vi "SIAM_test_Standalone-Dev.vi"() -> ()   [LabVIEW 2011]
doc: "Tool for TILL ID SIAM hardware test."
uses:
  SIAM_command.ctl
  SIAM-axis.ctl
  SIAM-send.ctl
panel:
  out "Connected":bool
  in  "Format":enum16{"Hex", "dez", "Ascii", "dez16s"}(ring)
  in  "Run":bool
  in  "Clear":bool
  in  "return":string
  in  "Registerkarte":T1(tab)
  in  "connect":bool caption="disconnect"
  in  "ScaleConst":T3(array[cluster])=[{"Axis-Ring"=104857665, "Scale"=500.0, "Offset"=1000000.0, "HW min"=0.0, "HW max"=4000.0, "max a"=inf, "max v"=inf, "units"="µm"}, {"Axis-Ring"=102760513, "Scale"=1.0, "Offset"=0.0, "HW min"=-32000.0, "HW max"=32000.0, "max a"=5.0, "max v"=inf, "units"="c"}, {"Axis-Ring"=101711937, "Scale"=1.0, "Offset"=0.0, "HW min"=-32000.0, "HW max"=32000.0, "max a"=0.02, "max v"=inf, "units"="c"}, {"Axis-Ring"=16777217, "Scale"=51200.0, "Offset"=100.0, "HW min"=0.0, "HW max"=5500000.0, "max a"=inf, "max v"=20.0, "units"="mm"}, {"Axis-Ring"=17825793, "Scale"=51200.0, "Offset"=100.0, "HW min"=0.0, "HW max"=3700000.0, "max a"=inf, "max v"=20.0, "units"="mm"}, {"Axis-Ring"=19922945, "Scale"=153600.0, "Offset"=146600.0, "HW min"=0.0, "HW max"=614400.0, "max a"=inf, "max v"=1.0, "units"="Pos"}, {"Axis-Ring"=20971521, "Scale"=25000.1, "Offset"=641.0, "HW min"=0.0, "HW max"=124721.0, "max a"=inf, "max v"=1.0, "units"="Pos"}, {"Axis-Ring"=22020097, "Scale"=1.0, "Offset"=0.0, "HW min"=0.0, "HW max"=51200.0, "max a"=inf, "max v"=inf, "units"="counts"}, {"Axis-Ring"=23068673, "Scale"=10240.0, "Offset"=0.0, "HW min"=0.0, "HW max"=51200.0, "max a"=inf, "max v"=inf, "units"="Pos"}, {"Axis-Ring"=24117249, "Scale"=1.0, "Offset"=0.0, "HW min"=0.0, "HW max"=51200.0, "max a"=inf, "max v"=inf, "units"="counts"}, {"Axis-Ring"=2684354561, "Scale"=1.0, "Offset"=0.0, "HW min"=0.0, "HW max"=65636.0, "max a"=inf, "max v"=inf, "units"="counts"}, {"Axis-Ring"=2685403137, "Scale"=1.0, "Offset"=0.0, "HW min"=0.0, "HW max"=65636.0, "max a"=inf, "max v"=inf, "units"="counts"}, {"Axis-Ring"=2686451713, "Scale"=1.0, "Offset"=0.0, "HW min"=0.0, "HW max"=65636.0, "max a"=inf, "max v"=inf, "units"="counts"}, {"Axis-Ring"=2687500289, "Scale"=1.0, "Offset"=0.0, "HW min"=0.0, "HW max"=65636.0, "max a"=inf, "max v"=inf, "units"="counts"}, {"Axis-Ring"=2688548865, "Scale"=1.0, "Offset"=0.0, "HW min"=0.0, "HW max"=65636.0, "max a"=inf, "max v"=inf, "units"="counts"}, {"Axis-Ring"=2689597441, "Scale"=1.0, "Offset"=1.0, "HW min"=0.0, "HW max"=65636.0, "max a"=inf, "max v"=inf, "units"="counts"}, {"Axis-Ring"=2690646017, "Scale"=1.0, "Offset"=1.0, "HW min"=0.0, "HW max"=65636.0, "max a"=inf, "max v"=inf, "units"="counts"}, {"Axis-Ring"=2691694593, "Scale"=1.0, "Offset"=1.0, "HW min"=0.0, "HW max"=65636.0, "max a"=inf, "max v"=inf, "units"="counts"}, {"Axis-Ring"=2701131777, "Scale"=1.0, "Offset"=1.0, "HW min"=0.0, "HW max"=65636.0, "max a"=inf, "max v"=inf, "units"="counts"}, {"Axis-Ring"=2702180353, "Scale"=1.0, "Offset"=1.0, "HW min"=0.0, "HW max"=65636.0, "max a"=inf, "max v"=inf, "units"="counts"}, {"Axis-Ring"=2703228929, "Scale"=1.0, "Offset"=1.0, "HW min"=0.0, "HW max"=65636.0, "max a"=inf, "max v"=inf, "units"="counts"}, {"Axis-Ring"=2704277505, "Scale"=1.0, "Offset"=1.0, "HW min"=0.0, "HW max"=65636.0, "max a"=inf, "max v"=inf, "units"="counts"}, {"Axis-Ring"=2717908993, "Scale"=1.0, "Offset"=1.0, "HW min"=0.0, "HW max"=65636.0, "max a"=inf, "max v"=inf, "units"="counts"}, {"Axis-Ring"=2718957569, "Scale"=1.0, "Offset"=1.0, "HW min"=0.0, "HW max"=65636.0, "max a"=inf, "max v"=inf, "units"="counts"}, {"Axis-Ring"=2720006145, "Scale"=1.0, "Offset"=1.0, "HW min"=0.0, "HW max"=65636.0, "max a"=inf, "max v"=inf, "units"="counts"}, {"Axis-Ring"=2721054721, "Scale"=1.0, "Offset"=1.0, "HW min"=0.0, "HW max"=65636.0, "max a"=inf, "max v"=inf, "units"="counts"}, {"Axis-Ring"=67108865, "Scale"=1.0, "Offset"=1.0, "HW min"=100000.0, "HW max"=200000.0, "max a"=inf, "max v"=inf, "units"="counts"}, {"Axis-Ring"=68157441, "Scale"=1.0, "Offset"=1.0, "HW min"=100000.0, "HW max"=200000.0, "max a"=inf, "max v"=inf, "units"="counts"}] {"Axis-Ring" items=["255Axis"=16777217, "1-Axis"=17825793, "2-Axis"=18874369, "3-Axis"=19922945, "4-Axis"=20971521, "5-Axis"=22020097, "6-Axis"=23068673, "7-Axis"=24117249, "LED365"=2684354561, "LED385"=2685403137, "LED440"=2686451713, "LED470"=2687500289, "LED510"=2688548865, "LED540"=2689597441, "LED590"=2690646017, "LED640"=2691694593, "DurchR"=2701131777, "DurchG"=2702180353, "DurchB"=2703228929, "AF"=2704277505, "Laser0"=2717908993, "Laser1"=2718957569, "Laser2"=2720006145, "Laser3"=2721054721, "Servo0"=67108865, "Servo1"=68157441, "Servo2"=69206017, "Servo3"=70254593, "0-TMSI"=100663361, "1-TMSI"=101711937, "x-tmsi"=102760513, "y-tmsi"=103809089, "z-tmsi"=104857665, "orca1"=503316481, "orca2"=503316482, "orca3"=503316483, "orca4"=503316484, ""=0]}
  in  "instrument name":string="Till-X-3"
  in  "remote port":u16=3
  in  "address":string="192.168.99.3"
  out "connect error":errorcluster
  in  "Read":bool
  in  "Axis":T4={"Linear"={"Axis-Ring"=17825793, "Position"=824034}, "Linear"={"Axis-Ring"=18874369, "Position"=463519}, "Linear 2"={"Axis-Ring"=19922945, "Position"=689614}, "Linear 3"={"Axis-Ring"=101711937, "Position"=0}, "Linear"={"Axis-Ring"=102760513, "Position"=0}, "Linear 4"={"Axis-Ring"=2684354561, "Position"=0}, "Linear 5"={"Axis-Ring"=2685403137, "Position"=0}, "Linear 6"={"Axis-Ring"=2687500289, "Position"=0}, "Linear 7"={"Axis-Ring"=2691694593, "Position"=0}, "Linear 8"={"Axis-Ring"=2701131777, "Position"=0}, "Linear 9"={"Axis-Ring"=2717908993, "Position"=0}, "Linear 10"={"Axis-Ring"=2718957569, "Position"=0}, "Linear 11"={"Axis-Ring"=2720006145, "Position"=0}, "Linear 12"={"Axis-Ring"=503316482, "Position"=0}, "Linear 13"={"Axis-Ring"=67108865, "Position"=150000}} {"Linear 13"."Axis-Ring" items=["X-Axis"=16777217, "Y-Axis"=17825793, "Obj"=19922945, "Filter"=20971521, "Trans"=22020097, "FRET"=23068673, "SI"=24117249, "LED365"=2684354561, "LED385"=2685403137, "LED440"=2686451713, "LED470"=2687500289, "LED510"=2688548865, "LED540"=2689597441, "LED590"=2690646017, "LED640"=2691694593, "DurchR"=2701131777, "DurchG"=2702180353, "DurchB"=2703228929, "AF"=2704277505, "Laser0"=2717908993, "Laser1"=2718957569, "Laser2"=2720006145, "Laser3"=2721054721, "Servo0"=67108865, "Servo1"=68157441, "Servo2"=69206017, "Servo3"=70254593]; "Linear 13"."Position" scale=100000.0..200000.0; "Linear 12"."Axis-Ring" items=["255Axis"=16777217, "1-Axis"=17825793, "2-Axis"=18874369, "3-Axis"=19922945, "4-Axis"=20971521, "5-Axis"=22020097, "6-Axis"=23068673, "7-Axis"=24117249, "LED365"=2684354561, "LED385"=2685403137, "LED440"=2686451713, "LED470"=2687500289, "LED510"=2688548865, "LED540"=2689597441, "LED590"=2690646017, "LED640"=2691694593, "DurchR"=2701131777, "DurchG"=2702180353, "DurchB"=2703228929, "AF"=2704277505, "Laser0"=2717908993, "Laser1"=2718957569, "Laser2"=2720006145, "Laser3"=2721054721, "Servo0"=67108865, "Servo1"=68157441, "Servo2"=69206017, "Servo3"=70254593, "0-TMSI"=100663361, "1-TMSI"=101711937, "x-tmsi"=102760513, "y-tmsi"=103809089, "z-tmsi"=104857665, "orca1"=503316481, "orca2"=503316482, "orca3"=503316483, "orca4"=503316484, ""=0]; "Linear 12"."Position" scale=0.0..100.0; "Linear 11"."Axis-Ring" items=["255Axis"=16777217, "1-Axis"=17825793, "2-Axis"=18874369, "3-Axis"=19922945, "4-Axis"=20971521, "5-Axis"=22020097, "6-Axis"=23068673, "7-Axis"=24117249, "LED365"=2684354561, "LED385"=2685403137, "LED440"=2686451713, "LED470"=2687500289, "LED510"=2688548865, "LED540"=2689597441, "LED590"=2690646017, "LED640"=2691694593, "DurchR"=2701131777, "DurchG"=2702180353, "DurchB"=2703228929, "AF"=2704277505, "Laser0"=2717908993, "Laser1"=2718957569, "Laser2"=2720006145, "Laser3"=2721054721, "Servo0"=67108865, "Servo1"=68157441, "Servo2"=69206017, "Servo3"=70254593, "0-TMSI"=100663361, "1-TMSI"=101711937, "x-tmsi"=102760513, "y-tmsi"=103809089, "z-tmsi"=104857665, "orca1"=503316481, "orca2"=503316482, "orca3"=503316483, "orca4"=503316484, ""=0]; "Linear 11"."Position" scale=0.0..65000.0; "Linear 10"."Axis-Ring" items=["255Axis"=16777217, "1-Axis"=17825793, "2-Axis"=18874369, "3-Axis"=19922945, "4-Axis"=20971521, "5-Axis"=22020097, "6-Axis"=23068673, "7-Axis"=24117249, "LED365"=2684354561, "LED385"=2685403137, "LED440"=2686451713, "LED470"=2687500289, "LED510"=2688548865, "LED540"=2689597441, "LED590"=2690646017, "LED640"=2691694593, "DurchR"=2701131777, "DurchG"=2702180353, "DurchB"=2703228929, "AF"=2704277505, "Laser0"=2717908993, "Laser1"=2718957569, "Laser2"=2720006145, "Laser3"=2721054721, "Servo0"=67108865, "Servo1"=68157441, "Servo2"=69206017, "Servo3"=70254593, "0-TMSI"=100663361, "1-TMSI"=101711937, "x-tmsi"=102760513, "y-tmsi"=103809089, "z-tmsi"=104857665, "orca1"=503316481, "orca2"=503316482, "orca3"=503316483, "orca4"=503316484, ""=0]; "Linear 10"."Position" scale=0.0..65000.0; "Linear 9"."Axis-Ring" items=["255Axis"=16777217, "1-Axis"=17825793, "2-Axis"=18874369, "3-Axis"=19922945, "4-Axis"=20971521, "5-Axis"=22020097, "6-Axis"=23068673, "7-Axis"=24117249, "LED365"=2684354561, "LED385"=2685403137, "LED440"=2686451713, "LED470"=2687500289, "LED510"=2688548865, "LED540"=2689597441, "LED590"=2690646017, "LED640"=2691694593, "DurchR"=2701131777, "DurchG"=2702180353, "DurchB"=2703228929, "AF"=2704277505, "Laser0"=2717908993, "Laser1"=2718957569, "Laser2"=2720006145, "Laser3"=2721054721, "Servo0"=67108865, "Servo1"=68157441, "Servo2"=69206017, "Servo3"=70254593, "0-TMSI"=100663361, "1-TMSI"=101711937, "x-tmsi"=102760513, "y-tmsi"=103809089, "z-tmsi"=104857665, "orca1"=503316481, "orca2"=503316482, "orca3"=503316483, "orca4"=503316484, ""=0]; "Linear 9"."Position" scale=0.0..65000.0; "Linear 8"."Axis-Ring" items=["255Axis"=16777217, "1-Axis"=17825793, "2-Axis"=18874369, "3-Axis"=19922945, "4-Axis"=20971521, "5-Axis"=22020097, "6-Axis"=23068673, "7-Axis"=24117249, "LED365"=2684354561, "LED385"=2685403137, "LED440"=2686451713, "LED470"=2687500289, "LED510"=2688548865, "LED540"=2689597441, "LED590"=2690646017, "LED640"=2691694593, "DurchR"=2701131777, "DurchG"=2702180353, "DurchB"=2703228929, "AF"=2704277505, "Laser0"=2717908993, "Laser1"=2718957569, "Laser2"=2720006145, "Laser3"=2721054721, "Servo0"=67108865, "Servo1"=68157441, "Servo2"=69206017, "Servo3"=70254593, "0-TMSI"=100663361, "1-TMSI"=101711937, "x-tmsi"=102760513, "y-tmsi"=103809089, "z-tmsi"=104857665, "orca1"=503316481, "orca2"=503316482, "orca3"=503316483, "orca4"=503316484, ""=0]; "Linear 8"."Position" scale=0.0..65000.0; "Linear 7"."Axis-Ring" items=["255Axis"=16777217, "1-Axis"=17825793, "2-Axis"=18874369, "3-Axis"=19922945, "4-Axis"=20971521, "5-Axis"=22020097, "6-Axis"=23068673, "7-Axis"=24117249, "LED365"=2684354561, "LED385"=2685403137, "LED440"=2686451713, "LED470"=2687500289, "LED510"=2688548865, "LED540"=2689597441, "LED590"=2690646017, "LED640"=2691694593, "DurchR"=2701131777, "DurchG"=2702180353, "DurchB"=2703228929, "AF"=2704277505, "Laser0"=2717908993, "Laser1"=2718957569, "Laser2"=2720006145, "Laser3"=2721054721, "Servo0"=67108865, "Servo1"=68157441, "Servo2"=69206017, "Servo3"=70254593, "0-TMSI"=100663361, "1-TMSI"=101711937, "x-tmsi"=102760513, "y-tmsi"=103809089, "z-tmsi"=104857665, "orca1"=503316481, "orca2"=503316482, "orca3"=503316483, "orca4"=503316484, ""=0]; "Linear 7"."Position" scale=0.0..65000.0; "Linear 6"."Axis-Ring" items=["255Axis"=16777217, "1-Axis"=17825793, "2-Axis"=18874369, "3-Axis"=19922945, "4-Axis"=20971521, "5-Axis"=22020097, "6-Axis"=23068673, "7-Axis"=24117249, "LED365"=2684354561, "LED385"=2685403137, "LED440"=2686451713, "LED470"=2687500289, "LED510"=2688548865, "LED540"=2689597441, "LED590"=2690646017, "LED640"=2691694593, "DurchR"=2701131777, "DurchG"=2702180353, "DurchB"=2703228929, "AF"=2704277505, "Laser0"=2717908993, "Laser1"=2718957569, "Laser2"=2720006145, "Laser3"=2721054721, "Servo0"=67108865, "Servo1"=68157441, "Servo2"=69206017, "Servo3"=70254593, "0-TMSI"=100663361, "1-TMSI"=101711937, "x-tmsi"=102760513, "y-tmsi"=103809089, "z-tmsi"=104857665, "orca1"=503316481, "orca2"=503316482, "orca3"=503316483, "orca4"=503316484, ""=0]; "Linear 6"."Position" scale=0.0..65000.0; "Linear 5"."Axis-Ring" items=["255Axis"=16777217, "1-Axis"=17825793, "2-Axis"=18874369, "3-Axis"=19922945, "4-Axis"=20971521, "5-Axis"=22020097, "6-Axis"=23068673, "7-Axis"=24117249, "LED365"=2684354561, "LED385"=2685403137, "LED440"=2686451713, "LED470"=2687500289, "LED510"=2688548865, "LED540"=2689597441, "LED590"=2690646017, "LED640"=2691694593, "DurchR"=2701131777, "DurchG"=2702180353, "DurchB"=2703228929, "AF"=2704277505, "Laser0"=2717908993, "Laser1"=2718957569, "Laser2"=2720006145, "Laser3"=2721054721, "Servo0"=67108865, "Servo1"=68157441, "Servo2"=69206017, "Servo3"=70254593, "0-TMSI"=100663361, "1-TMSI"=101711937, "x-tmsi"=102760513, "y-tmsi"=103809089, "z-tmsi"=104857665, "orca1"=503316481, "orca2"=503316482, "orca3"=503316483, "orca4"=503316484, ""=0]; "Linear 5"."Position" scale=0.0..65000.0; "Linear 4"."Axis-Ring" items=["255Axis"=16777217, "1-Axis"=17825793, "2-Axis"=18874369, "3-Axis"=19922945, "4-Axis"=20971521, "5-Axis"=22020097, "6-Axis"=23068673, "7-Axis"=24117249, "LED365"=2684354561, "LED385"=2685403137, "LED440"=2686451713, "LED470"=2687500289, "LED510"=2688548865, "LED540"=2689597441, "LED590"=2690646017, "LED640"=2691694593, "DurchR"=2701131777, "DurchG"=2702180353, "DurchB"=2703228929, "AF"=2704277505, "Laser0"=2717908993, "Laser1"=2718957569, "Laser2"=2720006145, "Laser3"=2721054721, "Servo0"=67108865, "Servo1"=68157441, "Servo2"=69206017, "Servo3"=70254593, "0-TMSI"=100663361, "1-TMSI"=101711937, "x-tmsi"=102760513, "y-tmsi"=103809089, "z-tmsi"=104857665, "orca1"=503316481, "orca2"=503316482, "orca3"=503316483, "orca4"=503316484, ""=0]; "Linear 4"."Position" scale=0.0..65000.0; "Linear"."Axis-Ring" items=["255Axis"=16777217, "1-Axis"=17825793, "2-Axis"=18874369, "3-Axis"=19922945, "4-Axis"=20971521, "5-Axis"=22020097, "6-Axis"=23068673, "7-Axis"=24117249, "LED365"=2684354561, "LED385"=2685403137, "LED440"=2686451713, "LED470"=2687500289, "LED510"=2688548865, "LED540"=2689597441, "LED590"=2690646017, "LED640"=2691694593, "DurchR"=2701131777, "DurchG"=2702180353, "DurchB"=2703228929, "AF"=2704277505, "Laser0"=2717908993, "Laser1"=2718957569, "Laser2"=2720006145, "Laser3"=2721054721, "Servo0"=67108865, "Servo1"=68157441, "Servo2"=69206017, "Servo3"=70254593, "0-TMSI"=100663361, "1-TMSI"=101711937, "x-tmsi"=102760513, "y-tmsi"=103809089, "z-tmsi"=104857665, "orca1"=503316481, "orca2"=503316482, "orca3"=503316483, "orca4"=503316484, ""=0]; "Linear"."Position" scale=-32000.0..32000.0; "Linear 3"."Axis-Ring" items=["255Axis"=16777217, "1-Axis"=17825793, "2-Axis"=18874369, "3-Axis"=19922945, "4-Axis"=20971521, "5-Axis"=22020097, "6-Axis"=23068673, "7-Axis"=24117249, "LED365"=2684354561, "LED385"=2685403137, "LED440"=2686451713, "LED470"=2687500289, "LED510"=2688548865, "LED540"=2689597441, "LED590"=2690646017, "LED640"=2691694593, "DurchR"=2701131777, "DurchG"=2702180353, "DurchB"=2703228929, "AF"=2704277505, "Laser0"=2717908993, "Laser1"=2718957569, "Laser2"=2720006145, "Laser3"=2721054721, "Servo0"=67108865, "Servo1"=68157441, "Servo2"=69206017, "Servo3"=70254593, "0-TMSI"=100663361, "1-TMSI"=101711937, "x-tmsi"=102760513, "y-tmsi"=103809089, "z-tmsi"=104857665, "orca1"=503316481, "orca2"=503316482, "orca3"=503316483, "orca4"=503316484, ""=0]; "Linear 3"."Position" scale=-32000.0..32000.0; "Linear 2"."Axis-Ring" items=["255Axis"=16777217, "1-Axis"=17825793, "2-Axis"=18874369, "3-Axis"=19922945, "4-Axis"=20971521, "5-Axis"=22020097, "6-Axis"=23068673, "7-Axis"=24117249, "LED365"=2684354561, "LED385"=2685403137, "LED440"=2686451713, "LED470"=2687500289, "LED510"=2688548865, "LED540"=2689597441, "LED590"=2690646017, "LED640"=2691694593, "DurchR"=2701131777, "DurchG"=2702180353, "DurchB"=2703228929, "AF"=2704277505, "Laser0"=2717908993, "Laser1"=2718957569, "Laser2"=2720006145, "Laser3"=2721054721, "Servo0"=67108865, "Servo1"=68157441, "Servo2"=69206017, "Servo3"=70254593, "0-TMSI"=100663361, "1-TMSI"=101711937, "x-tmsi"=102760513, "y-tmsi"=103809089, "z-tmsi"=104857665, "orca1"=503316481, "orca2"=503316482, "orca3"=503316483, "orca4"=503316484, ""=0]; "Linear 2"."Position" scale=-100000.0..50000.0; "Linear"."Axis-Ring" items=["255Axis"=16777217, "1-Axis"=17825793, "2-Axis"=18874369, "3-Axis"=19922945, "4-Axis"=20971521, "5-Axis"=22020097, "6-Axis"=23068673, "7-Axis"=24117249, "LED365"=2684354561, "LED385"=2685403137, "LED440"=2686451713, "LED470"=2687500289, "LED510"=2688548865, "LED540"=2689597441, "LED590"=2690646017, "LED640"=2691694593, "DurchR"=2701131777, "DurchG"=2702180353, "DurchB"=2703228929, "AF"=2704277505, "Laser0"=2717908993, "Laser1"=2718957569, "Laser2"=2720006145, "Laser3"=2721054721, "Servo0"=67108865, "Servo1"=68157441, "Servo2"=69206017, "Servo3"=70254593, "0-TMSI"=100663361, "1-TMSI"=101711937, "x-tmsi"=102760513, "y-tmsi"=103809089, "z-tmsi"=104857665, "orca1"=503316481, "orca2"=503316482, "orca3"=503316483, "orca4"=503316484, ""=0]; "Linear"."Position" scale=-250000.0..250000.0; "Linear"."Axis-Ring" items=["255Axis"=16777217, "1-Axis"=17825793, "2-Axis"=18874369, "3-Axis"=19922945, "4-Axis"=20971521, "5-Axis"=22020097, "6-Axis"=23068673, "7-Axis"=24117249, "LED365"=2684354561, "LED385"=2685403137, "LED440"=2686451713, "LED470"=2687500289, "LED510"=2688548865, "LED540"=2689597441, "LED590"=2690646017, "LED640"=2691694593, "DurchR"=2701131777, "DurchG"=2702180353, "DurchB"=2703228929, "AF"=2704277505, "Laser0"=2717908993, "Laser1"=2718957569, "Laser2"=2720006145, "Laser3"=2721054721, "Servo0"=67108865, "Servo1"=68157441, "Servo2"=69206017, "Servo3"=70254593, "0-TMSI"=100663361, "1-TMSI"=101711937, "x-tmsi"=102760513, "y-tmsi"=103809089, "z-tmsi"=104857665, "orca1"=503316481, "orca2"=503316482, "orca3"=503316483, "orca4"=503316484, ""=0]; "Linear"."Position" scale=-1024000.0..1024000.0}
  in  "Array":T5(array[cluster])=[{"Digital-out"=enum."cam1", "Boolean"=FALSE}, {"Digital-out"=enum."cam2", "Boolean"=FALSE}, {"Digital-out"=enum."led2", "Boolean"=FALSE}, {"Digital-out"=enum."led3", "Boolean"=FALSE}, {"Digital-out"=enum."led4", "Boolean"=FALSE}, {"Digital-out"=enum."led5", "Boolean"=FALSE}, {"Digital-out"=enum."led5", "Boolean"=FALSE}, {"Digital-out"=enum."led7", "Boolean"=FALSE}, {"Digital-out"=enum."led8", "Boolean"=FALSE}, {"Digital-out"=enum."durchR", "Boolean"=FALSE}, {"Digital-out"=enum."tsm-pwr", "Boolean"=FALSE}, {"Digital-out"=enum."dc-pwr", "Boolean"=FALSE}, {"Digital-out"=enum."laser-pwr", "Boolean"=FALSE}, {"Digital-out"=enum."Laser0", "Boolean"=FALSE}, {"Digital-out"=enum."Laser1", "Boolean"=FALSE}, {"Digital-out"=enum."Laser2", "Boolean"=FALSE}, {"Digital-out"=enum."Laser3", "Boolean"=FALSE}, {"Digital-out"=enum."TrigOut", "Boolean"=FALSE}, {"Digital-out"=enum."SMB1", "Boolean"=FALSE}]
  in  "xy":T6
  in  "step":i32=42345
  in  "Calculate SIM":bool
  out "Camera":T7={"Camera-Expos ms"=0.0, "CameraImages"=7, "cam fps min."=0.0}
  in  "Constants":T9={"galvox-Line0"=14814, "GalvoX-Blanking"=15000.0, "galvox-count/pix"=-2.474, "Camera-StartLine"=-62, "Camera-Endline"=4000, "Wobbel-total"=4280.0, "SM_ticks"=20, "Trigger_ticks"=100, "galvoxAccel"=5.0, "WobbelAccel"=0.01, "zAccel"=0.05, "z-delay-ticks"=700, "SCMOS-LineSpeed [10µs]"=2.4996, "RS height- Pix"=100, "extra-xgalvo"=83.0, "zcommand"=4026531840, "min turn ticks"=500.0} {"zcommand" format="%x" items=["end_no_ticket"=4027514895, "end_ticket"=4027518991, "NoOp"=4026531840, "Read ticks"=4026535936, "Read ticks to var"=4026535938, "Read IP"=4043313152, "Read IP into var"=4043313154, "Set IP from var"=4043309059, "Set IP from var, relative"=4043313155, "branchRel_if_equal"=4043374849, "decrement_branchRel_if_equal"=4043374945, "decrement_branchRel_if_greaterequal"=4043375201, "decrement_branchRel_if_greaterequal_withTicket"=4043379297, "decrement_branchRel_if_smaller"=4043375457, "increment_branchRel_if_smaller"=4043375473, "readVar"=4060090368, "writeVar"=4060086273, "copyVar0_from_var1"=4060086275, "math_addToVariable"=4076863488, "math_addVToVariable"=4076863489, "math_subToVariable"=4076863490, "math_subVToVariable"=4076863491, "math_multToVariable"=4076863492, "math_multvToVariable"=4076863493, "math_divideToVariable"=4076863494, "math_divideVToVariable"=4076863495, "math_modToVariable"=4076863496, "math_modVToVariable"=4076863497, "logic_and"=4093640704, "logic_or"=4093640706, "logic_xor"=4093640708, "bitshift"=4093640712, "I2C-write"=335544337, "I2C-read"=335548433, "Cam-SPI-write"=3254779905, "UART0-VC-Baud-write"=469958673, "UART0-VC-Baud-read"=469962768, "UART0-VC-write"=469762065, "UART0-VC-write-Var"=469762067, "UART0-VC-read-availabe-bytes-to-var"=470355970, "UART0-VC-read-availabe-bytes"=470355984, "UART0-VC-read-skip-bytes"=469831681, "UART0-VC-read"=469766160, "UART0-VC-read-Var"=469766162, "UART1-TSM-Baud-write"=486735889, "UART1-TSM-Baud-read"=486739984, "UART1-TSM-write"=486539281, "UART1-TSM-write-Var"=486539283, "UART1-TSM-read-availabe-bytes-to-var"=487133186, "UART1-TSM-read-availabe-bytes"=487133200, "UART1-TSM-read-skip-bytes"=486604801, "UART1-TSM-read-skip-bytes"=486608897, "UART1-TSM-read"=486543376, "UART1-TSM-read-Var"=486543378, "UART2-Laser-Baud-write"=503513105, "UART2-Baud-read"=503517200, "UART2-write"=503316497, "UART2-write-Var"=503316499, "UART2-read-availabe-bytes-to-var"=503910402, "UART2-read-availabe-bytes"=503910416, "UART2-read-skip-bytes"=503386113, "UART2-read"=503320592, "UART2-read-Var"=503320594, "UART3-Baud-write"=520290321, "UART3-Baud-read"=520294416, "UART3-write"=520093713, "UART3-write-Var"=520093715, "UART3-read-availabe-bytes-to-var"=520687618, "UART3-read-availabe-bytes"=520687632, "UART3-read-skip-bytes"=520163329, "UART3-read"=520097808, "UART3-read-Var"=520097810, "IO-read_bank0"=3489665024, "IO-write_bank0"=3489660929, "IO-read_bank1"=3506442240, "IO-write_bank1"=3506438145, "DA0-0_LED365"=2684354561, "DA0-1_LED385"=2685403137, "DA0-2_LED440"=2686451713, "DA0-3_LED470"=2687500289, "DA0-4_LED510"=2688548865, "DA0-5_LED550"=2689597441, "DA0-6_LED590"=2690646017, "DA0-7_LED640"=2691694593, "DA1-0_LED-R"=2701131777, "DA1-1_LED-G"=2702180353, "DA1-2_LED-B"=2703228929, "DA1-3_LED-AF"=2704277505, "DA1-4"=2705326081, "DA1-5"=2706374657, "DA1-6"=2707423233, "DA1-7"=2708471809, "DA2-Laser0"=2717908993, "DA2-Laser1"=2718957569, "DA2-Laser2"=2720006145, "DA2-Laser3"=2721054721, "DA2-Laser4"=2722103297, "Analog-read_AD0-0"=2818576384, "Analog-read-store_AD0-0"=2818572290, "AF-Register-transfer r/w"=2835349505, "AF-Register-read"=2835353600, "AF-Register-read-to-var"=2835353602, "AF-Transfer-from-var"=2835349507, "IO-delay_bank0"=3489923073, "IO-delay_bank0_fromVar"=3489923075, "read_cam_clock"=3289124864, "store_cam_clock"=3289120770, "read_cam_phase"=3289190400, "store_cam_phase"=3289186306, "store_cam_phase-t"=3289190402, "r_cam1_NHS"=3254980608, "w_cam1_NHS"=3254976513, "r_cam1_NVS"=3255046144, "w_cam1_NVS"=3255042049, "r_cam1_npx"=3255111680, "w_cam1_npx"=3255107585, "r_cam1_npy"=3255177216, "w_cam1_npy"=3255173121, "r_cam1_xhswait"=3255439360, "w_cam1_xhswait"=3255435265, "r_cam1_xvs_wait"=3255504896, "w_cam1_xvs_wait"=3255500801, "r_cam1_framcounter"=3255570432, "r_cam1_line"=3255635968, "r_cam1_xhs-counter"=3255701504, "r_cam2_NHS"=3271757824, "w_cam2_NHS"=3271753729, "r_cam2_NVS"=3271823360, "w_cam2_NVS"=3271819265, "r_cam2_npx"=3271888896, "w_cam2_npx"=3271884801, "r_cam2_npy"=3271954432, "w_cam2_npy"=3271950337, "r_cam2_xvs_wait"=3272282112, "w_cam2_xvs_wait"=3272278017, "r_cam2_framcounter"=3272347648, "r_cam2_line"=3272413184, "r_cam2_xhs-counter"=3272478720, "start TMSI"=102694919, "set_1Galvo"=101712113, "set_x-Galvo"=102760689, "set_y-Galvo"=103809265, "set_z-Fokus"=104857841, "set_1Galvo_position-only"=101711937, "set_x-Galvo_position-only"=102760513, "set_y-Galvo_position-only"=103809089, "set_z-Fokus_position-only"=104857665, "set_x-Galvo_position-only_ticket"=102764609, "set_y-Galvo_position-only_ticket"=103813185, "set_z-Fokus_position-only_ticket"=104861761, "set_1Galvo_relativ-only"=101712001, "set_x-Galvo_relativ-only"=102760577, "set_y-Galvo_relativ-only"=103809153, "set_z-Fokus_relativ-only"=104857729, "set_1Galvo_speed-only"=101711905, "set_x-Galvo_speed-only"=102760481, "set_y-Galvo_speed-only"=103809057, "set_z-Fokus_speed-only"=104857633, "set_1Galvo_acc-only"=101711889, "set_x-Galvo_acc-only"=102760465, "set_y-Galvo_acc-only"=103809041, "set_z-Fokus_acc-only"=104857617, "read_1Galvo_ticket"=101716032, "read_x-Galvo_ticket"=102764608, "read_y-Galvo_ticket"=103813184, "read_z-Focus_ticket"=104861760, "x-Galvo_pos_fromVar"=102760515, "y-Galvo_pos_fromVar"=103809091, "z-Focus_pos_fromVar"=104857667, "Servo0"=67108865, "Servo0-enable"=68091911, "Servo0-disable"=68091919, "Servo1"=68157441, "Servo1-enable"=69140487, "Servo1-disable"=69140495, "Servo2-enable"=70189063, "Servo2"=69206017, "Servo3-enable"=71237639, "Servo3"=70254593, "x-ssi-init"=202309639, "x-ssi-disable"=202309647, "x-ssi-Bits"=201523201, "x-ssi-Read"=201330688, "x-ssi-ReadToVar"=201326594, "x-ssi-ReadToVar-ticket"=201330690, "y-ssi-init"=203358215, "y-ssi-disable"=203358223, "y-ssi-Bits"=202571777, "y-ssi-Read"=202379264, "y-ssi-ReadToVar"=202375170, "y-ssi-ReadToVat-ticket"=202379266]; "SCMOS-LineSpeed [10µs]" format="%#.6f" items=["EdgeFast-285MHz"=0.9175, "EdgeSlow-95MHz"=2.7525, "Panda4.2"=2.7766, "mer2000-12"=2.4996, "mer2000-8bit"=1.25]; "galvox-count/pix" format="%#_5f"}
  in  "User":T10={"z-distance_motorunits"=100, "#planes"=1, "Digital-out"=enum."Laser1", "NoOfPhaseImages"=7} {"#planes" min=1}
  in  "SendScript":bool
  in  "Load":bool
  in  "Save":bool
  in  "ClearScript":bool
  in  "Script":T11(array[cluster])=[{"Delay 10µs"=0, "command"=4027514895, "P0"=0, "P1"=0, "P2"=0, "P3"=0, "P4"=0, "P5-ticket"=0, "comment"=""}] {"command" format="%x" items=["end_no_ticket"=4027514895, "end_ticket"=4027518991, "NoOp"=4026531840, "Read ticks"=4026535936, "Read ticks to var"=4026535938, "Read IP"=4043313152, "Read IP into var"=4043313154, "Set IP from var"=4043309059, "Set IP from var, relative"=4043313155, "branchRel_if_equal"=4043374849, "decrement_branchRel_if_equal"=4043374945, "decrement_branchRel_if_greaterequal"=4043375201, "decrement_branchRel_if_greaterequal_withTicket"=4043379297, "decrement_branchRel_if_smaller"=4043375457, "increment_branchRel_if_smaller"=4043375473, "readVar"=4060090368, "writeVar"=4060086273, "copyVar0_from_var1"=4060086275, "math_addToVariable"=4076863488, "math_addVToVariable"=4076863489, "math_subToVariable"=4076863490, "math_subVToVariable"=4076863491, "math_multToVariable"=4076863492, "math_multvToVariable"=4076863493, "math_divideToVariable"=4076863494, "math_divideVToVariable"=4076863495, "math_modToVariable"=4076863496, "math_modVToVariable"=4076863497, "logic_and"=4093640704, "logic_or"=4093640706, "logic_xor"=4093640708, "bitshift"=4093640712, "I2C-write"=335544337, "I2C-read"=335548433, "Cam-SPI-write"=3254779905, "UART0-VC-Baud-write"=469958673, "UART0-VC-Baud-read"=469962768, "UART0-VC-write"=469762065, "UART0-VC-write-Var"=469762067, "UART0-VC-read-availabe-bytes-to-var"=470355970, "UART0-VC-read-availabe-bytes"=470355984, "UART0-VC-read-skip-bytes"=469831681, "UART0-VC-read"=469766160, "UART0-VC-read-Var"=469766162, "UART1-TSM-Baud-write"=486735889, "UART1-TSM-Baud-read"=486739984, "UART1-TSM-write"=486539281, "UART1-TSM-write-Var"=486539283, "UART1-TSM-read-availabe-bytes-to-var"=487133186, "UART1-TSM-read-availabe-bytes"=487133200, "UART1-TSM-read-skip-bytes"=486604801, "UART1-TSM-read-skip-bytes"=486608897, "UART1-TSM-read"=486543376, "UART1-TSM-read-Var"=486543378, "UART2-Laser-Baud-write"=503513105, "UART2-Baud-read"=503517200, "UART2-write"=503316497, "UART2-write-Var"=503316499, "UART2-read-availabe-bytes-to-var"=503910402, "UART2-read-availabe-bytes"=503910416, "UART2-read-skip-bytes"=503386113, "UART2-read"=503320592, "UART2-read-Var"=503320594, "UART3-Baud-write"=520290321, "UART3-Baud-read"=520294416, "UART3-write"=520093713, "UART3-write-Var"=520093715, "UART3-read-availabe-bytes-to-var"=520687618, "UART3-read-availabe-bytes"=520687632, "UART3-read-skip-bytes"=520163329, "UART3-read"=520097808, "UART3-read-Var"=520097810, "IO-read_bank0"=3489665024, "IO-write_bank0"=3489660929, "IO-read_bank1"=3506442240, "IO-write_bank1"=3506438145, "DA0-0_LED365"=2684354561, "DA0-1_LED385"=2685403137, "DA0-2_LED440"=2686451713, "DA0-3_LED470"=2687500289, "DA0-4_LED510"=2688548865, "DA0-5_LED550"=2689597441, "DA0-6_LED590"=2690646017, "DA0-7_LED640"=2691694593, "DA1-0_LED-R"=2701131777, "DA1-1_LED-G"=2702180353, "DA1-2_LED-B"=2703228929, "DA1-3_LED-AF"=2704277505, "DA1-4"=2705326081, "DA1-5"=2706374657, "DA1-6"=2707423233, "DA1-7"=2708471809, "DA2-Laser0"=2717908993, "DA2-Laser1"=2718957569, "DA2-Laser2"=2720006145, "DA2-Laser3"=2721054721, "DA2-Laser4"=2722103297, "Analog-read_AD0-0"=2818576384, "Analog-read-store_AD0-0"=2818572290, "AF-Register-transfer r/w"=2835349505, "AF-Register-read"=2835353600, "AF-Register-read-to-var"=2835353602, "AF-Transfer-from-var"=2835349507, "IO-delay_bank0"=3489923073, "IO-delay_bank0_fromVar"=3489923075, "read_cam_clock"=3289124864, "store_cam_clock"=3289120770, "read_cam_phase"=3289190400, "store_cam_phase"=3289186306, "store_cam_phase-t"=3289190402, "r_cam1_NHS"=3254980608, "w_cam1_NHS"=3254976513, "r_cam1_NVS"=3255046144, "w_cam1_NVS"=3255042049, "r_cam1_npx"=3255111680, "w_cam1_npx"=3255107585, "r_cam1_npy"=3255177216, "w_cam1_npy"=3255173121, "r_cam1_xhswait"=3255439360, "w_cam1_xhswait"=3255435265, "r_cam1_xvs_wait"=3255504896, "w_cam1_xvs_wait"=3255500801, "r_cam1_framcounter"=3255570432, "r_cam1_line"=3255635968, "r_cam1_xhs-counter"=3255701504, "r_cam2_NHS"=3271757824, "w_cam2_NHS"=3271753729, "r_cam2_NVS"=3271823360, "w_cam2_NVS"=3271819265, "r_cam2_npx"=3271888896, "w_cam2_npx"=3271884801, "r_cam2_npy"=3271954432, "w_cam2_npy"=3271950337, "r_cam2_xvs_wait"=3272282112, "w_cam2_xvs_wait"=3272278017, "r_cam2_framcounter"=3272347648, "r_cam2_line"=3272413184, "r_cam2_xhs-counter"=3272478720, "start TMSI"=102694919, "set_1Galvo"=101712113, "set_x-Galvo"=102760689, "set_y-Galvo"=103809265, "set_z-Fokus"=104857841, "set_1Galvo_position-only"=101711937, "set_x-Galvo_position-only"=102760513, "set_y-Galvo_position-only"=103809089, "set_z-Fokus_position-only"=104857665, "set_x-Galvo_position-only_ticket"=102764609, "set_y-Galvo_position-only_ticket"=103813185, "set_z-Fokus_position-only_ticket"=104861761, "set_1Galvo_relativ-only"=101712001, "set_x-Galvo_relativ-only"=102760577, "set_y-Galvo_relativ-only"=103809153, "set_z-Fokus_relativ-only"=104857729, "set_1Galvo_speed-only"=101711905, "set_x-Galvo_speed-only"=102760481, "set_y-Galvo_speed-only"=103809057, "set_z-Fokus_speed-only"=104857633, "set_1Galvo_acc-only"=101711889, "set_x-Galvo_acc-only"=102760465, "set_y-Galvo_acc-only"=103809041, "set_z-Fokus_acc-only"=104857617, "read_1Galvo_ticket"=101716032, "read_x-Galvo_ticket"=102764608, "read_y-Galvo_ticket"=103813184, "read_z-Focus_ticket"=104861760, "x-Galvo_pos_fromVar"=102760515, "y-Galvo_pos_fromVar"=103809091, "z-Focus_pos_fromVar"=104857667, "Servo0"=67108865, "Servo0-enable"=68091911, "Servo0-disable"=68091919, "Servo1"=68157441, "Servo1-enable"=69140487, "Servo1-disable"=69140495, "Servo2-enable"=70189063, "Servo2"=69206017, "Servo3-enable"=71237639, "Servo3"=70254593, "x-ssi-init"=202309639, "x-ssi-disable"=202309647, "x-ssi-Bits"=201523201, "x-ssi-Read"=201330688, "x-ssi-ReadToVar"=201326594, "x-ssi-ReadToVar-ticket"=201330690, "y-ssi-init"=203358215, "y-ssi-disable"=203358223, "y-ssi-Bits"=202571777, "y-ssi-Read"=202379264, "y-ssi-ReadToVar"=202375170, "y-ssi-ReadToVat-ticket"=202379266]; "P5-ticket" format="%.0x"; "Delay 10µs" format="%.0x"; "P0" format="%.0x"; "P1" format="%.0x"}
  in  "Clear direct":bool
  in  "UART: 0..3":u8=2 max=3
  in  "Uart-TSM":bool
  in  "Uart-Ascii":bool
  in  "Special":bool
  in  "direkt command queue":T11(array[cluster])=[{"Delay 10µs"=0, "command"=102694919, "P0"=0, "P1"=0, "P2"=0, "P3"=0, "P4"=0, "P5-ticket"=0, "comment"=""}] {"command" format="%x" items=["end_no_ticket"=4027514895, "end_ticket"=4027518991, "NoOp"=4026531840, "Read ticks"=4026535936, "Read ticks to var"=4026535938, "Read IP"=4043313152, "Read IP into var"=4043313154, "Set IP from var"=4043309059, "Set IP from var, relative"=4043313155, "branchRel_if_equal"=4043374849, "decrement_branchRel_if_equal"=4043374945, "decrement_branchRel_if_greaterequal"=4043375201, "decrement_branchRel_if_greaterequal_withTicket"=4043379297, "decrement_branchRel_if_smaller"=4043375457, "increment_branchRel_if_smaller"=4043375473, "readVar"=4060090368, "writeVar"=4060086273, "copyVar0_from_var1"=4060086275, "math_addToVariable"=4076863488, "math_addVToVariable"=4076863489, "math_subToVariable"=4076863490, "math_subVToVariable"=4076863491, "math_multToVariable"=4076863492, "math_multvToVariable"=4076863493, "math_divideToVariable"=4076863494, "math_divideVToVariable"=4076863495, "math_modToVariable"=4076863496, "math_modVToVariable"=4076863497, "logic_and"=4093640704, "logic_or"=4093640706, "logic_xor"=4093640708, "bitshift"=4093640712, "I2C-write"=335544337, "I2C-read"=335548433, "Cam-SPI-write"=3254779905, "UART0-VC-Baud-write"=469958673, "UART0-VC-Baud-read"=469962768, "UART0-VC-write"=469762065, "UART0-VC-write-Var"=469762067, "UART0-VC-read-availabe-bytes-to-var"=470355970, "UART0-VC-read-availabe-bytes"=470355984, "UART0-VC-read-skip-bytes"=469831681, "UART0-VC-read"=469766160, "UART0-VC-read-Var"=469766162, "UART1-TSM-Baud-write"=486735889, "UART1-TSM-Baud-read"=486739984, "UART1-TSM-write"=486539281, "UART1-TSM-write-Var"=486539283, "UART1-TSM-read-availabe-bytes-to-var"=487133186, "UART1-TSM-read-availabe-bytes"=487133200, "UART1-TSM-read-skip-bytes"=486604801, "UART1-TSM-read-skip-bytes"=486608897, "UART1-TSM-read"=486543376, "UART1-TSM-read-Var"=486543378, "UART2-Laser-Baud-write"=503513105, "UART2-Baud-read"=503517200, "UART2-write"=503316497, "UART2-write-Var"=503316499, "UART2-read-availabe-bytes-to-var"=503910402, "UART2-read-availabe-bytes"=503910416, "UART2-read-skip-bytes"=503386113, "UART2-read"=503320592, "UART2-read-Var"=503320594, "UART3-Baud-write"=520290321, "UART3-Baud-read"=520294416, "UART3-write"=520093713, "UART3-write-Var"=520093715, "UART3-read-availabe-bytes-to-var"=520687618, "UART3-read-availabe-bytes"=520687632, "UART3-read-skip-bytes"=520163329, "UART3-read"=520097808, "UART3-read-Var"=520097810, "IO-read_bank0"=3489665024, "IO-write_bank0"=3489660929, "IO-read_bank1"=3506442240, "IO-write_bank1"=3506438145, "DA0-0_LED365"=2684354561, "DA0-1_LED385"=2685403137, "DA0-2_LED440"=2686451713, "DA0-3_LED470"=2687500289, "DA0-4_LED510"=2688548865, "DA0-5_LED550"=2689597441, "DA0-6_LED590"=2690646017, "DA0-7_LED640"=2691694593, "DA1-0_LED-R"=2701131777, "DA1-1_LED-G"=2702180353, "DA1-2_LED-B"=2703228929, "DA1-3_LED-AF"=2704277505, "DA1-4"=2705326081, "DA1-5"=2706374657, "DA1-6"=2707423233, "DA1-7"=2708471809, "DA2-Laser0"=2717908993, "DA2-Laser1"=2718957569, "DA2-Laser2"=2720006145, "DA2-Laser3"=2721054721, "DA2-Laser4"=2722103297, "Analog-read_AD0-0"=2818576384, "Analog-read-store_AD0-0"=2818572290, "AF-Register-transfer r/w"=2835349505, "AF-Register-read"=2835353600, "AF-Register-read-to-var"=2835353602, "AF-Transfer-from-var"=2835349507, "IO-delay_bank0"=3489923073, "IO-delay_bank0_fromVar"=3489923075, "read_cam_clock"=3289124864, "store_cam_clock"=3289120770, "read_cam_phase"=3289190400, "store_cam_phase"=3289186306, "store_cam_phase-t"=3289190402, "r_cam1_NHS"=3254980608, "w_cam1_NHS"=3254976513, "r_cam1_NVS"=3255046144, "w_cam1_NVS"=3255042049, "r_cam1_npx"=3255111680, "w_cam1_npx"=3255107585, "r_cam1_npy"=3255177216, "w_cam1_npy"=3255173121, "r_cam1_xhswait"=3255439360, "w_cam1_xhswait"=3255435265, "r_cam1_xvs_wait"=3255504896, "w_cam1_xvs_wait"=3255500801, "r_cam1_framcounter"=3255570432, "r_cam1_line"=3255635968, "r_cam1_xhs-counter"=3255701504, "r_cam2_NHS"=3271757824, "w_cam2_NHS"=3271753729, "r_cam2_NVS"=3271823360, "w_cam2_NVS"=3271819265, "r_cam2_npx"=3271888896, "w_cam2_npx"=3271884801, "r_cam2_npy"=3271954432, "w_cam2_npy"=3271950337, "r_cam2_xvs_wait"=3272282112, "w_cam2_xvs_wait"=3272278017, "r_cam2_framcounter"=3272347648, "r_cam2_line"=3272413184, "r_cam2_xhs-counter"=3272478720, "start TMSI"=102694919, "set_1Galvo"=101712113, "set_x-Galvo"=102760689, "set_y-Galvo"=103809265, "set_z-Fokus"=104857841, "set_1Galvo_position-only"=101711937, "set_x-Galvo_position-only"=102760513, "set_y-Galvo_position-only"=103809089, "set_z-Fokus_position-only"=104857665, "set_x-Galvo_position-only_ticket"=102764609, "set_y-Galvo_position-only_ticket"=103813185, "set_z-Fokus_position-only_ticket"=104861761, "set_1Galvo_relativ-only"=101712001, "set_x-Galvo_relativ-only"=102760577, "set_y-Galvo_relativ-only"=103809153, "set_z-Fokus_relativ-only"=104857729, "set_1Galvo_speed-only"=101711905, "set_x-Galvo_speed-only"=102760481, "set_y-Galvo_speed-only"=103809057, "set_z-Fokus_speed-only"=104857633, "set_1Galvo_acc-only"=101711889, "set_x-Galvo_acc-only"=102760465, "set_y-Galvo_acc-only"=103809041, "set_z-Fokus_acc-only"=104857617, "read_1Galvo_ticket"=101716032, "read_x-Galvo_ticket"=102764608, "read_y-Galvo_ticket"=103813184, "read_z-Focus_ticket"=104861760, "x-Galvo_pos_fromVar"=102760515, "y-Galvo_pos_fromVar"=103809091, "z-Focus_pos_fromVar"=104857667, "Servo0"=67108865, "Servo0-enable"=68091911, "Servo0-disable"=68091919, "Servo1"=68157441, "Servo1-enable"=69140487, "Servo1-disable"=69140495, "Servo2-enable"=70189063, "Servo2"=69206017, "Servo3-enable"=71237639, "Servo3"=70254593, "x-ssi-init"=202309639, "x-ssi-disable"=202309647, "x-ssi-Bits"=201523201, "x-ssi-Read"=201330688, "x-ssi-ReadToVar"=201326594, "x-ssi-ReadToVar-ticket"=201330690, "y-ssi-init"=203358215, "y-ssi-disable"=203358223, "y-ssi-Bits"=202571777, "y-ssi-Read"=202379264, "y-ssi-ReadToVar"=202375170, "y-ssi-ReadToVat-ticket"=202379266]; "P5-ticket" format="%.0x"; "P0" format="%.0x"; "P2" format="%.0x"; "P1" format="%.0x"}
  in  "TSM":T12={"RS232-axis"=255, "axis"=255, "Command"="?TILL_STATUS", "value"=946.0} {"RS232-axis" format="%0d"}
  in  "String":string(combo)="SOUR2:POW:LEV:IMM:AMPL?\r"
  in  "Wait ms":i32=500
  in  "direkt commands":T11(array[cluster])=[{"Delay 10µs"=0, "command"=102694919, "P0"=0, "P1"=0, "P2"=0, "P3"=0, "P4"=0, "P5-ticket"=0, "comment"=""}] {"command" format="%x" items=["end_no_ticket"=4027514895, "end_ticket"=4027518991, "NoOp"=4026531840, "Read ticks"=4026535936, "Read ticks to var"=4026535938, "Read IP"=4043313152, "Read IP into var"=4043313154, "Set IP from var"=4043309059, "Set IP from var, relative"=4043313155, "branchRel_if_equal"=4043374849, "decrement_branchRel_if_equal"=4043374945, "decrement_branchRel_if_greaterequal"=4043375201, "decrement_branchRel_if_greaterequal_withTicket"=4043379297, "decrement_branchRel_if_smaller"=4043375457, "increment_branchRel_if_smaller"=4043375473, "readVar"=4060090368, "writeVar"=4060086273, "copyVar0_from_var1"=4060086275, "math_addToVariable"=4076863488, "math_addVToVariable"=4076863489, "math_subToVariable"=4076863490, "math_subVToVariable"=4076863491, "math_multToVariable"=4076863492, "math_multvToVariable"=4076863493, "math_divideToVariable"=4076863494, "math_divideVToVariable"=4076863495, "math_modToVariable"=4076863496, "math_modVToVariable"=4076863497, "logic_and"=4093640704, "logic_or"=4093640706, "logic_xor"=4093640708, "bitshift"=4093640712, "I2C-write"=335544337, "I2C-read"=335548433, "Cam-SPI-write"=3254779905, "UART0-VC-Baud-write"=469958673, "UART0-VC-Baud-read"=469962768, "UART0-VC-write"=469762065, "UART0-VC-write-Var"=469762067, "UART0-VC-read-availabe-bytes-to-var"=470355970, "UART0-VC-read-availabe-bytes"=470355984, "UART0-VC-read-skip-bytes"=469831681, "UART0-VC-read"=469766160, "UART0-VC-read-Var"=469766162, "UART1-TSM-Baud-write"=486735889, "UART1-TSM-Baud-read"=486739984, "UART1-TSM-write"=486539281, "UART1-TSM-write-Var"=486539283, "UART1-TSM-read-availabe-bytes-to-var"=487133186, "UART1-TSM-read-availabe-bytes"=487133200, "UART1-TSM-read-skip-bytes"=486604801, "UART1-TSM-read-skip-bytes"=486608897, "UART1-TSM-read"=486543376, "UART1-TSM-read-Var"=486543378, "UART2-Laser-Baud-write"=503513105, "UART2-Baud-read"=503517200, "UART2-write"=503316497, "UART2-write-Var"=503316499, "UART2-read-availabe-bytes-to-var"=503910402, "UART2-read-availabe-bytes"=503910416, "UART2-read-skip-bytes"=503386113, "UART2-read"=503320592, "UART2-read-Var"=503320594, "UART3-Baud-write"=520290321, "UART3-Baud-read"=520294416, "UART3-write"=520093713, "UART3-write-Var"=520093715, "UART3-read-availabe-bytes-to-var"=520687618, "UART3-read-availabe-bytes"=520687632, "UART3-read-skip-bytes"=520163329, "UART3-read"=520097808, "UART3-read-Var"=520097810, "IO-read_bank0"=3489665024, "IO-write_bank0"=3489660929, "IO-read_bank1"=3506442240, "IO-write_bank1"=3506438145, "DA0-0_LED365"=2684354561, "DA0-1_LED385"=2685403137, "DA0-2_LED440"=2686451713, "DA0-3_LED470"=2687500289, "DA0-4_LED510"=2688548865, "DA0-5_LED550"=2689597441, "DA0-6_LED590"=2690646017, "DA0-7_LED640"=2691694593, "DA1-0_LED-R"=2701131777, "DA1-1_LED-G"=2702180353, "DA1-2_LED-B"=2703228929, "DA1-3_LED-AF"=2704277505, "DA1-4"=2705326081, "DA1-5"=2706374657, "DA1-6"=2707423233, "DA1-7"=2708471809, "DA2-Laser0"=2717908993, "DA2-Laser1"=2718957569, "DA2-Laser2"=2720006145, "DA2-Laser3"=2721054721, "DA2-Laser4"=2722103297, "Analog-read_AD0-0"=2818576384, "Analog-read-store_AD0-0"=2818572290, "AF-Register-transfer r/w"=2835349505, "AF-Register-read"=2835353600, "AF-Register-read-to-var"=2835353602, "AF-Transfer-from-var"=2835349507, "IO-delay_bank0"=3489923073, "IO-delay_bank0_fromVar"=3489923075, "read_cam_clock"=3289124864, "store_cam_clock"=3289120770, "read_cam_phase"=3289190400, "store_cam_phase"=3289186306, "store_cam_phase-t"=3289190402, "r_cam1_NHS"=3254980608, "w_cam1_NHS"=3254976513, "r_cam1_NVS"=3255046144, "w_cam1_NVS"=3255042049, "r_cam1_npx"=3255111680, "w_cam1_npx"=3255107585, "r_cam1_npy"=3255177216, "w_cam1_npy"=3255173121, "r_cam1_xhswait"=3255439360, "w_cam1_xhswait"=3255435265, "r_cam1_xvs_wait"=3255504896, "w_cam1_xvs_wait"=3255500801, "r_cam1_framcounter"=3255570432, "r_cam1_line"=3255635968, "r_cam1_xhs-counter"=3255701504, "r_cam2_NHS"=3271757824, "w_cam2_NHS"=3271753729, "r_cam2_NVS"=3271823360, "w_cam2_NVS"=3271819265, "r_cam2_npx"=3271888896, "w_cam2_npx"=3271884801, "r_cam2_npy"=3271954432, "w_cam2_npy"=3271950337, "r_cam2_xvs_wait"=3272282112, "w_cam2_xvs_wait"=3272278017, "r_cam2_framcounter"=3272347648, "r_cam2_line"=3272413184, "r_cam2_xhs-counter"=3272478720, "start TMSI"=102694919, "set_1Galvo"=101712113, "set_x-Galvo"=102760689, "set_y-Galvo"=103809265, "set_z-Fokus"=104857841, "set_1Galvo_position-only"=101711937, "set_x-Galvo_position-only"=102760513, "set_y-Galvo_position-only"=103809089, "set_z-Fokus_position-only"=104857665, "set_x-Galvo_position-only_ticket"=102764609, "set_y-Galvo_position-only_ticket"=103813185, "set_z-Fokus_position-only_ticket"=104861761, "set_1Galvo_relativ-only"=101712001, "set_x-Galvo_relativ-only"=102760577, "set_y-Galvo_relativ-only"=103809153, "set_z-Fokus_relativ-only"=104857729, "set_1Galvo_speed-only"=101711905, "set_x-Galvo_speed-only"=102760481, "set_y-Galvo_speed-only"=103809057, "set_z-Fokus_speed-only"=104857633, "set_1Galvo_acc-only"=101711889, "set_x-Galvo_acc-only"=102760465, "set_y-Galvo_acc-only"=103809041, "set_z-Fokus_acc-only"=104857617, "read_1Galvo_ticket"=101716032, "read_x-Galvo_ticket"=102764608, "read_y-Galvo_ticket"=103813184, "read_z-Focus_ticket"=104861760, "x-Galvo_pos_fromVar"=102760515, "y-Galvo_pos_fromVar"=103809091, "z-Focus_pos_fromVar"=104857667, "Servo0"=67108865, "Servo0-enable"=68091911, "Servo0-disable"=68091919, "Servo1"=68157441, "Servo1-enable"=69140487, "Servo1-disable"=69140495, "Servo2-enable"=70189063, "Servo2"=69206017, "Servo3-enable"=71237639, "Servo3"=70254593, "x-ssi-init"=202309639, "x-ssi-disable"=202309647, "x-ssi-Bits"=201523201, "x-ssi-Read"=201330688, "x-ssi-ReadToVar"=201326594, "x-ssi-ReadToVar-ticket"=201330690, "y-ssi-init"=203358215, "y-ssi-disable"=203358223, "y-ssi-Bits"=202571777, "y-ssi-Read"=202379264, "y-ssi-ReadToVar"=202375170, "y-ssi-ReadToVat-ticket"=202379266]; "P5-ticket" format="%.0x"; "P0" format="%.0x"; "P2" format="%.0x"; "P1" format="%.0x"}
  out "init error":errorcluster
  in  "New Ini":bool
  in  "end-read":bool
  out "Return":i32[](array[numeric])=[120, 0] format="%.0x"
  out "send error":errorcluster
  out "recieve error":errorcluster
  out "connection ID":refnum<k5>
  out "Send debug":T11(array[cluster]) {"command" format="%x" items=["end_no_ticket"=4027514895, "end_ticket"=4027518991, "NoOp"=4026531840, "Read ticks"=4026535936, "Read ticks to var"=4026535938, "Read IP"=4043313152, "Read IP into var"=4043313154, "Set IP from var"=4043309059, "Set IP from var, relative"=4043313155, "branchRel_if_equal"=4043374849, "decrement_branchRel_if_equal"=4043374945, "decrement_branchRel_if_greaterequal"=4043375201, "decrement_branchRel_if_greaterequal_withTicket"=4043379297, "decrement_branchRel_if_smaller"=4043375457, "increment_branchRel_if_smaller"=4043375473, "readVar"=4060090368, "writeVar"=4060086273, "copyVar0_from_var1"=4060086275, "math_addToVariable"=4076863488, "math_addVToVariable"=4076863489, "math_subToVariable"=4076863490, "math_subVToVariable"=4076863491, "math_multToVariable"=4076863492, "math_multvToVariable"=4076863493, "math_divideToVariable"=4076863494, "math_divideVToVariable"=4076863495, "math_modToVariable"=4076863496, "math_modVToVariable"=4076863497, "logic_and"=4093640704, "logic_or"=4093640706, "logic_xor"=4093640708, "bitshift"=4093640712, "I2C-write"=335544337, "I2C-read"=335548433, "Cam-SPI-write"=3254779905, "UART0-VC-Baud-write"=469958673, "UART0-VC-Baud-read"=469962768, "UART0-VC-write"=469762065, "UART0-VC-write-Var"=469762067, "UART0-VC-read-availabe-bytes-to-var"=470355970, "UART0-VC-read-availabe-bytes"=470355984, "UART0-VC-read-skip-bytes"=469831681, "UART0-VC-read"=469766160, "UART0-VC-read-Var"=469766162, "UART1-TSM-Baud-write"=486735889, "UART1-TSM-Baud-read"=486739984, "UART1-TSM-write"=486539281, "UART1-TSM-write-Var"=486539283, "UART1-TSM-read-availabe-bytes-to-var"=487133186, "UART1-TSM-read-availabe-bytes"=487133200, "UART1-TSM-read-skip-bytes"=486604801, "UART1-TSM-read-skip-bytes"=486608897, "UART1-TSM-read"=486543376, "UART1-TSM-read-Var"=486543378, "UART2-Laser-Baud-write"=503513105, "UART2-Baud-read"=503517200, "UART2-write"=503316497, "UART2-write-Var"=503316499, "UART2-read-availabe-bytes-to-var"=503910402, "UART2-read-availabe-bytes"=503910416, "UART2-read-skip-bytes"=503386113, "UART2-read"=503320592, "UART2-read-Var"=503320594, "UART3-Baud-write"=520290321, "UART3-Baud-read"=520294416, "UART3-write"=520093713, "UART3-write-Var"=520093715, "UART3-read-availabe-bytes-to-var"=520687618, "UART3-read-availabe-bytes"=520687632, "UART3-read-skip-bytes"=520163329, "UART3-read"=520097808, "UART3-read-Var"=520097810, "IO-read_bank0"=3489665024, "IO-write_bank0"=3489660929, "IO-read_bank1"=3506442240, "IO-write_bank1"=3506438145, "DA0-0_LED365"=2684354561, "DA0-1_LED385"=2685403137, "DA0-2_LED440"=2686451713, "DA0-3_LED470"=2687500289, "DA0-4_LED510"=2688548865, "DA0-5_LED550"=2689597441, "DA0-6_LED590"=2690646017, "DA0-7_LED640"=2691694593, "DA1-0_LED-R"=2701131777, "DA1-1_LED-G"=2702180353, "DA1-2_LED-B"=2703228929, "DA1-3_LED-AF"=2704277505, "DA1-4"=2705326081, "DA1-5"=2706374657, "DA1-6"=2707423233, "DA1-7"=2708471809, "DA2-Laser0"=2717908993, "DA2-Laser1"=2718957569, "DA2-Laser2"=2720006145, "DA2-Laser3"=2721054721, "DA2-Laser4"=2722103297, "Analog-read_AD0-0"=2818576384, "Analog-read-store_AD0-0"=2818572290, "AF-Register-transfer r/w"=2835349505, "AF-Register-read"=2835353600, "AF-Register-read-to-var"=2835353602, "AF-Transfer-from-var"=2835349507, "IO-delay_bank0"=3489923073, "IO-delay_bank0_fromVar"=3489923075, "read_cam_clock"=3289124864, "store_cam_clock"=3289120770, "read_cam_phase"=3289190400, "store_cam_phase"=3289186306, "store_cam_phase-t"=3289190402, "r_cam1_NHS"=3254980608, "w_cam1_NHS"=3254976513, "r_cam1_NVS"=3255046144, "w_cam1_NVS"=3255042049, "r_cam1_npx"=3255111680, "w_cam1_npx"=3255107585, "r_cam1_npy"=3255177216, "w_cam1_npy"=3255173121, "r_cam1_xhswait"=3255439360, "w_cam1_xhswait"=3255435265, "r_cam1_xvs_wait"=3255504896, "w_cam1_xvs_wait"=3255500801, "r_cam1_framcounter"=3255570432, "r_cam1_line"=3255635968, "r_cam1_xhs-counter"=3255701504, "r_cam2_NHS"=3271757824, "w_cam2_NHS"=3271753729, "r_cam2_NVS"=3271823360, "w_cam2_NVS"=3271819265, "r_cam2_npx"=3271888896, "w_cam2_npx"=3271884801, "r_cam2_npy"=3271954432, "w_cam2_npy"=3271950337, "r_cam2_xvs_wait"=3272282112, "w_cam2_xvs_wait"=3272278017, "r_cam2_framcounter"=3272347648, "r_cam2_line"=3272413184, "r_cam2_xhs-counter"=3272478720, "start TMSI"=102694919, "set_1Galvo"=101712113, "set_x-Galvo"=102760689, "set_y-Galvo"=103809265, "set_z-Fokus"=104857841, "set_1Galvo_position-only"=101711937, "set_x-Galvo_position-only"=102760513, "set_y-Galvo_position-only"=103809089, "set_z-Fokus_position-only"=104857665, "set_x-Galvo_position-only_ticket"=102764609, "set_y-Galvo_position-only_ticket"=103813185, "set_z-Fokus_position-only_ticket"=104861761, "set_1Galvo_relativ-only"=101712001, "set_x-Galvo_relativ-only"=102760577, "set_y-Galvo_relativ-only"=103809153, "set_z-Fokus_relativ-only"=104857729, "set_1Galvo_speed-only"=101711905, "set_x-Galvo_speed-only"=102760481, "set_y-Galvo_speed-only"=103809057, "set_z-Fokus_speed-only"=104857633, "set_1Galvo_acc-only"=101711889, "set_x-Galvo_acc-only"=102760465, "set_y-Galvo_acc-only"=103809041, "set_z-Fokus_acc-only"=104857617, "read_1Galvo_ticket"=101716032, "read_x-Galvo_ticket"=102764608, "read_y-Galvo_ticket"=103813184, "read_z-Focus_ticket"=104861760, "x-Galvo_pos_fromVar"=102760515, "y-Galvo_pos_fromVar"=103809091, "z-Focus_pos_fromVar"=104857667, "Servo0"=67108865, "Servo0-enable"=68091911, "Servo0-disable"=68091919, "Servo1"=68157441, "Servo1-enable"=69140487, "Servo1-disable"=69140495, "Servo2-enable"=70189063, "Servo2"=69206017, "Servo3-enable"=71237639, "Servo3"=70254593, "x-ssi-init"=202309639, "x-ssi-disable"=202309647, "x-ssi-Bits"=201523201, "x-ssi-Read"=201330688, "x-ssi-ReadToVar"=201326594, "x-ssi-ReadToVar-ticket"=201330690, "y-ssi-init"=203358215, "y-ssi-disable"=203358223, "y-ssi-Bits"=202571777, "y-ssi-Read"=202379264, "y-ssi-ReadToVar"=202375170, "y-ssi-ReadToVat-ticket"=202379266]; "P5-ticket" format="%.0x"; "Delay 10µs" format="%.0x"; "P0" format="%.0x"; "P1" format="%.0x"}
  out "Ini-file used":path
  in  "wrapper[U32]":u32[](array[ring])=[67] format="%x" items=["p-Stop"=112, "1-ReInit FPGA"=49, "C-Clear Error"=67, "d-Dump registers"=100, "r-Read register"=114, "D-Dump memory"=68, "t-run"=116, "w-Write"=119]
  in  "Wrapper":bool
  in  "End":bool
  # "better this scales, for each device? - So far not implememted\ne.g Galvo +-30°opt,f=50mm: 7.9897E-7 m/count"
  # "ring has to match command!"
  # "HW=val*scale+offset  (also offset ist in hardwareunits)(time in v,a in s or 10µs units?)"
  # "scale    offset   min max maxa maxv  name"
  # "todo: read+update"
  # "Neu: Parabolic!"
  # "read cam: e.g. AC076=704630 \n(/256/100)=27.5246µs"
  # "alles umgestellt auf count und Pixel und 10µs !!!"
  # "shift full phase"
  # "software timing"
  # "0: dcc22\n1: technosoft\n2: laser\n3: dc1000, usb,thermo"
  # "cr=\\r\nlf=\\n"
  # "16bit is shiftetd to msb (*65536)"
  # "todo: TSM other than UART1"
  # "MSR [6E81]: upd,Event,On,x/reached,contour,complete,trigger/LSN,LSP,wrap,x/err,SW,upd-Err,Init\nMER [0]: Off,CommErr,UV,OV, OT-d,OT-m,I2T,OC,LSN,LSP,Wrap,SerialE,ContE,Setup,short,CAN"
  # "version 20220216"
  # "logger for special tickets???"
  # "21.7.2020\nvalues are now array"
  # "update values if exsiting"
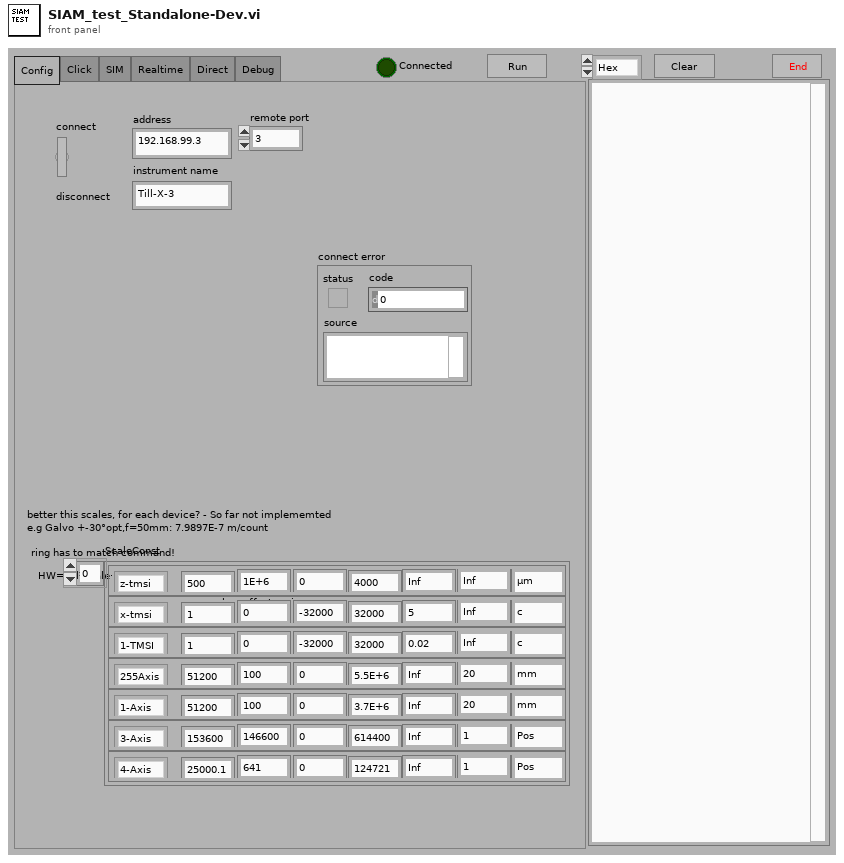
[diagram p1: front panel]
types:
  T1 = enum32{"Config", "Click", "SIM", "Realtime", "Direct", "Debug"}
  T2 = typedef "SIAM-axis.ctl" = u32
  T3 = cluster{"Axis-Ring":T2, "Scale":dbl, "Offset":dbl, "HW min":dbl, "HW max":dbl, "max a":dbl, "max v":dbl, "units":string}[]
  T4 = cluster{"Linear":cluster{"Axis-Ring":T2, "Position":i32}, "Linear":cluster{"Axis-Ring":T2, "Position":i32}, "Linear 2":cluster{"Axis-Ring":T2, "Position":i32}, "Linear 3":cluster{"Axis-Ring":T2, "Position":i32}, "Linear":cluster{"Axis-Ring":T2, "Position":i32}, "Linear 4":cluster{"Axis-Ring":T2, "Position":i32}, "Linear 5":cluster{"Axis-Ring":T2, "Position":i32}, "Linear 6":cluster{"Axis-Ring":T2, "Position":i32}, "Linear 7":cluster{"Axis-Ring":T2, "Position":i32}, "Linear 8":cluster{"Axis-Ring":T2, "Position":i32}, "Linear 9":cluster{"Axis-Ring":T2, "Position":i32}, "Linear 10":cluster{"Axis-Ring":T2, "Position":i32}, "Linear 11":cluster{"Axis-Ring":T2, "Position":i32}, "Linear 12":cluster{"Axis-Ring":T2, "Position":i32}, "Linear 13":cluster{"Axis-Ring":u32, "Position":i32}}
  T5 = cluster{"Digital-out":enum8{"cam1", "cam1-ready?", "cam2", "cam2-ready?", "tmsx?", "tsmy?", "tsm3?", "lid?", "led1", "led2", "led3", "led4", "led5", "led6", "led7", "led8", "durchR", "tsm-pwr", "dc-pwr", "laser-pwr", "Laser0", "Laser1", "Laser2", "Laser3", "Laser4", "LaserX", "TrigOut", "SMB1", ""}, "Boolean":bool}[]
  T6 = cluster{"x":bool, "y":bool, "-x":bool, "-y":bool}
  T7 = cluster{"Camera-Expos ms":dbl, "CameraImages":u16, "cam fps min.":dbl}
  T8 = typedef "SIAM_command.ctl" = u32
  T9 = cluster{"galvox-Line0":i16, "GalvoX-Blanking":dbl, "galvox-count/pix":dbl, "Camera-StartLine":i32, "Camera-Endline":u32, "Wobbel-total":dbl, "SM_ticks":u32, "Trigger_ticks":u32, "galvoxAccel":dbl, "WobbelAccel":dbl, "zAccel":dbl, "z-delay-ticks":u32, "SCMOS-LineSpeed [10µs]":dbl, "RS height- Pix":u16, "extra-xgalvo":dbl, "zcommand":T8, "min turn ticks":dbl}
  T10 = cluster{"z-distance_motorunits":i32, "#planes":u16, "Digital-out":enum8{"cam1", "cam1-ready?", "cam2", "cam2-ready?", "tmsx?", "tsmy?", "tsm3?", "lid?", "led1", "led2", "led3", "led4", "led5", "led6", "led7", "led8", "durchR", "durchG", "durchB", "AF", "Laser0", "Laser1", "Laser2", "Laser3", "Laser4", "LaserX", "TrigOut", "SMB1", ""}, "NoOfPhaseImages":u16}
  T11 = cluster{"Delay 10µs":u32, "command":T8, "P0":i32, "P1":i32, "P2":i32, "P3":i32, "P4":i32, "P5-ticket":i32, "comment":string}[]
  T12 = cluster{"RS232-axis":u8, "axis":u8, "Command":string, "value":dbl}
  T13 = enum16{"Standard", "Buffered", "CRLF", "Immediate"}
  T14 = typedef "SIAM-send.ctl" = enum16{"validID", "storeID", "enable", "rundirect", "sendlist", "run", "stop", "readRegister", "sendValue", "storeStatus"}
  T15 = cluster{"Delay 10µs":u32, "command":T8, "P0":i32, "P1":i32, "P2":i32, "P3":i32, "P4":i32, "P5-ticket":i32, string}[]
  T16 = cluster{"rel 10µs":u32, "Device":T8, "data0":i32, "data1":i32, "data2":i32, "data3":i32, "data4":i32, "data5":i32, string}
  T17 = cluster{"Delay 10µs":u32, "command":T8, "P0":i32, "P1":i32, "P2":i32, "P3":i32, "P4":i32, "P5-ticket":i32, "comment":string}
  T18 = enum8{"cam1", "cam1-ready?", "cam2", "cam2-ready?", "tmsx?", "tsmy?", "tsm3?", "lid?", "led1", "led2", "led3", "led4", "led5", "led6", "led7", "led8", "durchR", "tsm-pwr", "dc-pwr", "laser-pwr", "Laser0", "Laser1", "Laser2", "Laser3", "Laser4", "LaserX", "TrigOut", "SMB1", ""}
  T19 = cluster{"rel 10µs":u32, "Device":T8, "data0":i32, "data1":i32, "data2":i32, "data3":i32, "data4":i32, "data5":i32, string}[]
  T20 = cluster{"Delay 10µs":u32, "command":T8, "P0":i32, "P1":i32, "P2":i32, "P3":i32, "P4":i32, "P5-ticket":i32, "Comment":string}[]
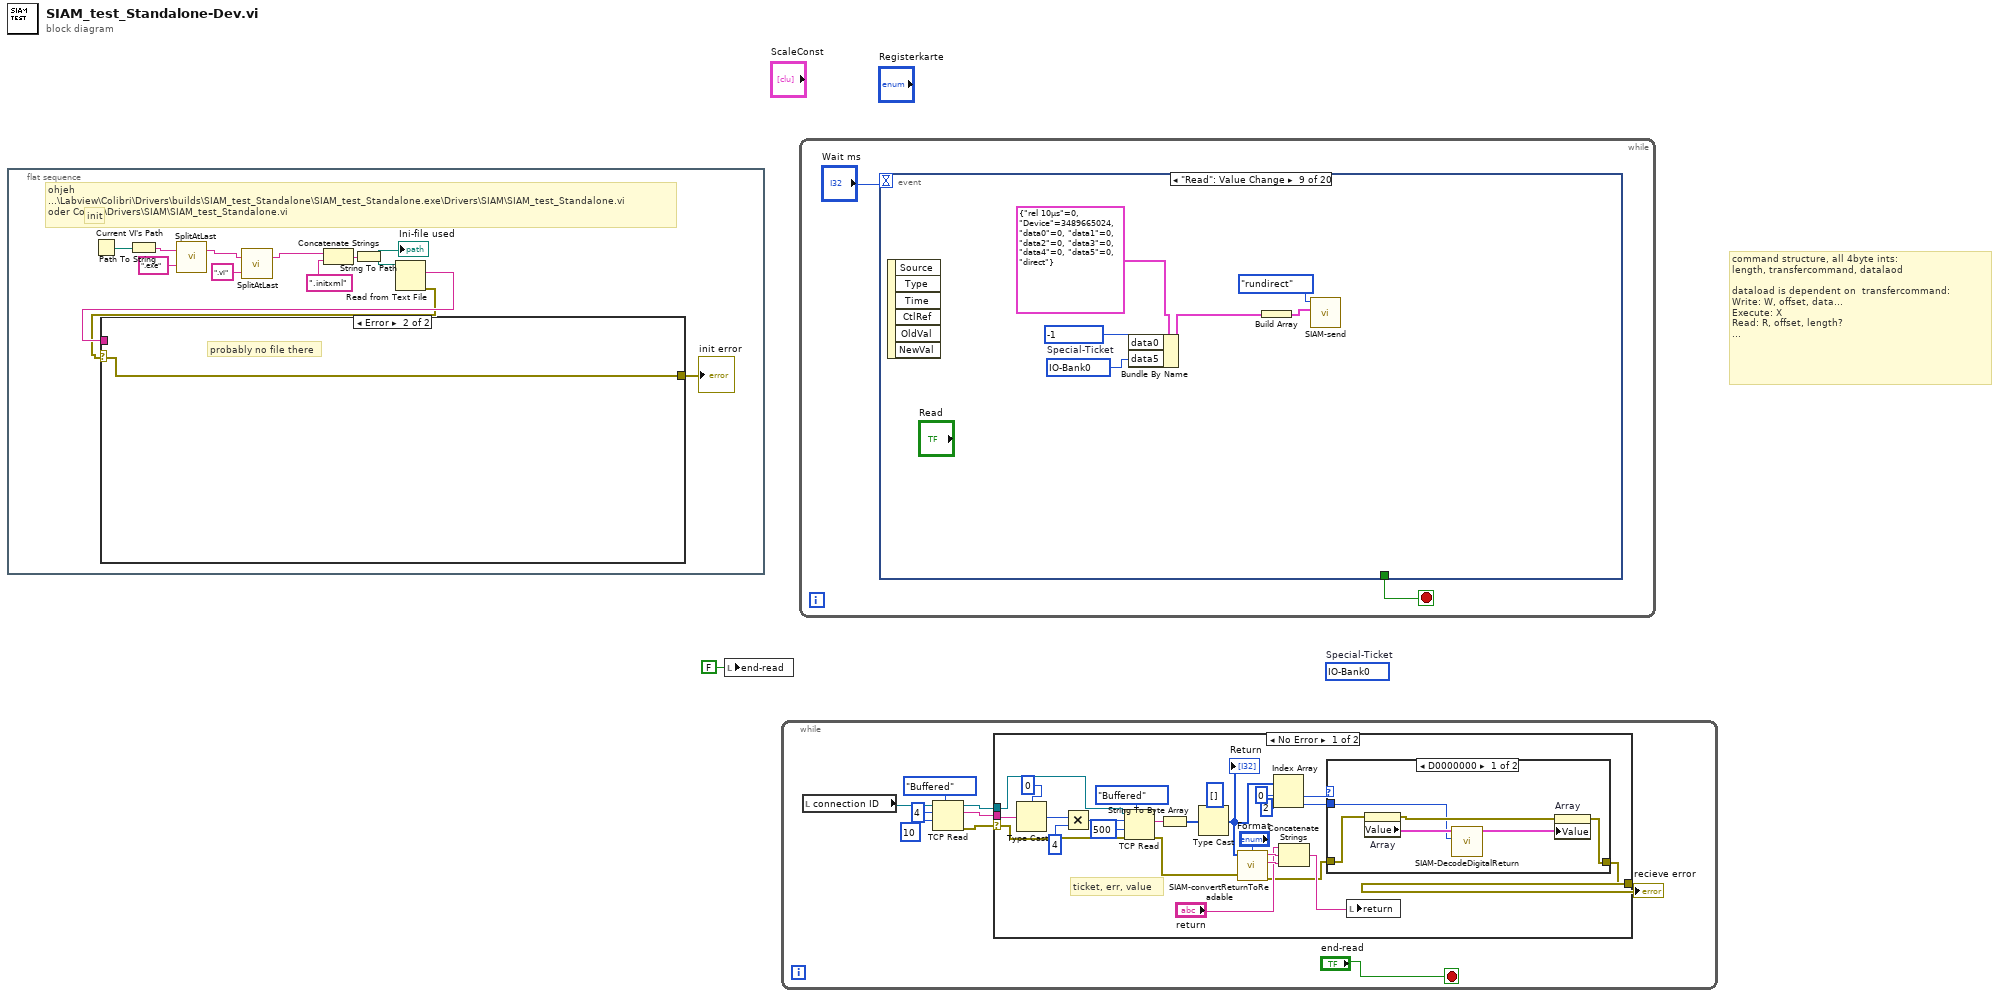
[diagram p0: block diagram]
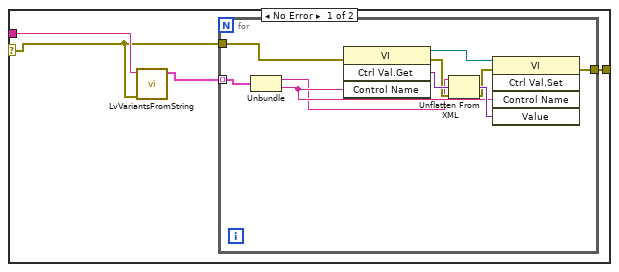
[diagram p2: hidden frame]
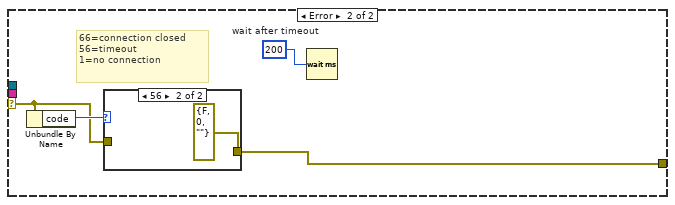
[diagram p4: hidden frame]
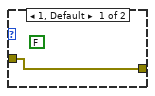
[diagram p5: hidden frame]
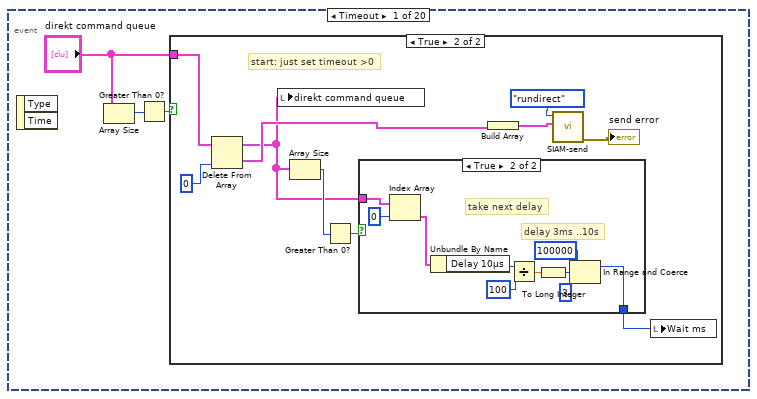
[diagram p6: hidden frame]
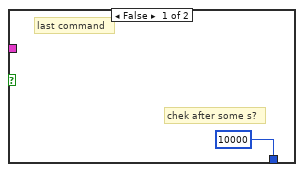
[diagram p8: hidden frame]
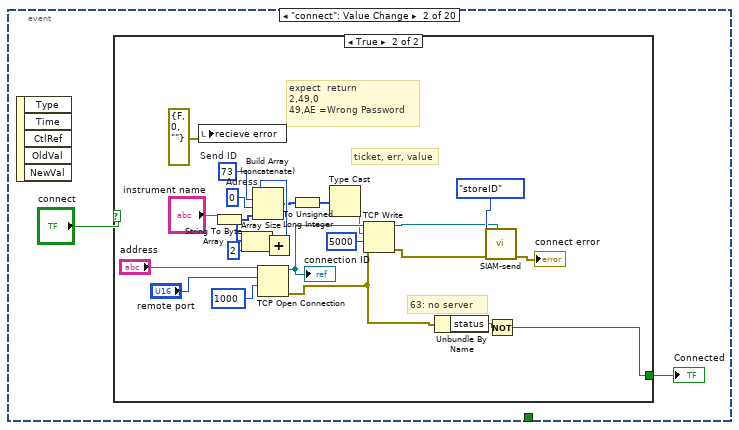
[diagram p9: hidden frame]
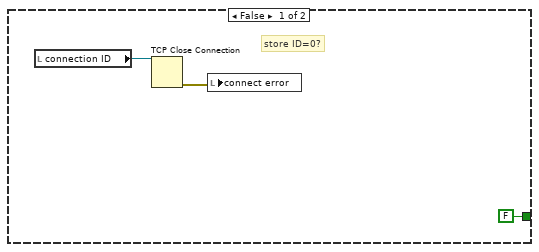
[diagram p10: hidden frame]
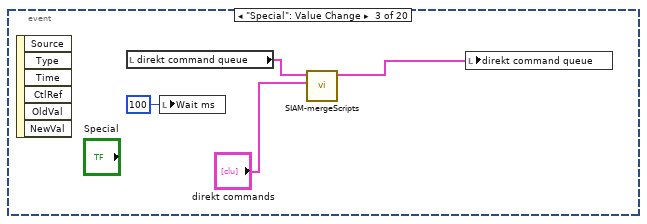
[diagram p11: hidden frame]
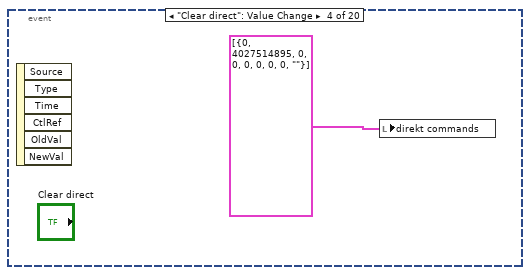
[diagram p12: hidden frame]
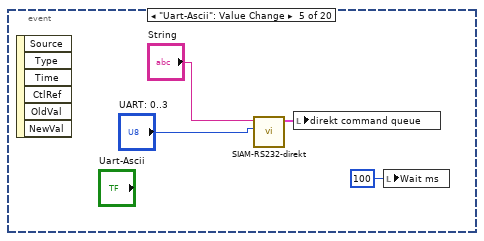
[diagram p13: hidden frame]
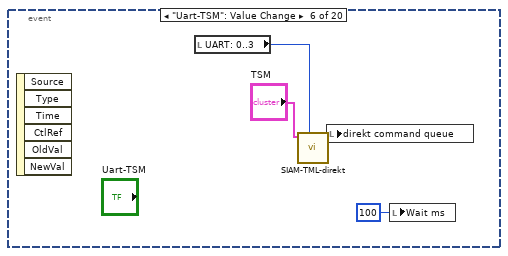
[diagram p14: hidden frame]
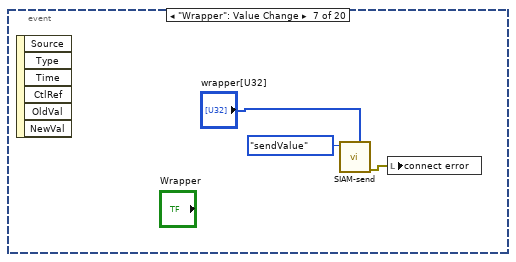
[diagram p15: hidden frame]
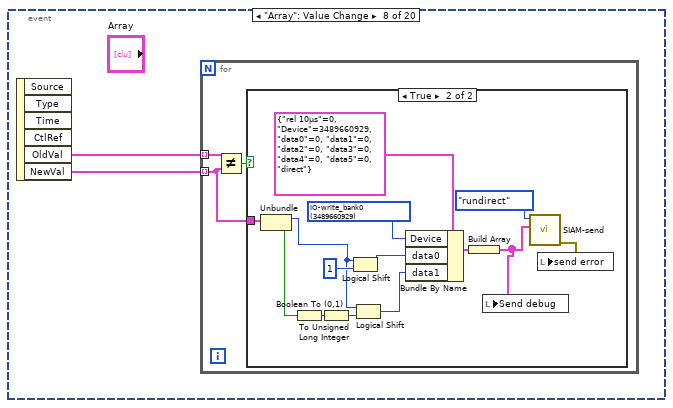
[diagram p16: hidden frame]
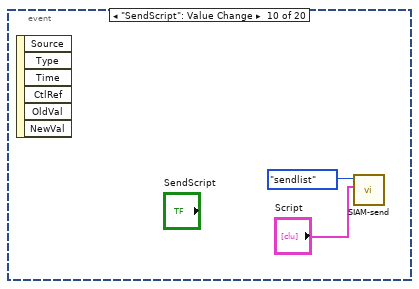
[diagram p18: hidden frame]
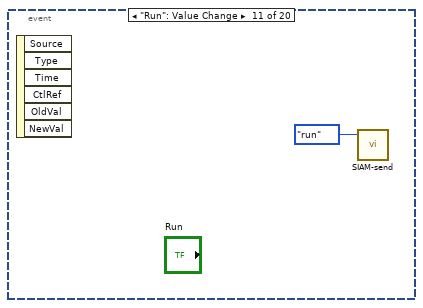
[diagram p19: hidden frame]
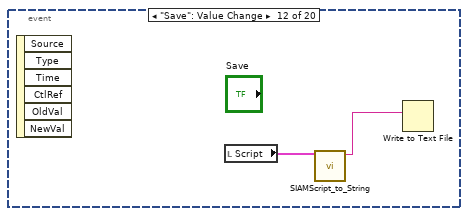
[diagram p20: hidden frame]
diagram:
  (unwired) T2 3489660928 items=["255Axis"=16777217, "1-Axis"=17825793, "2-Axis"=18874369, "3-Axis"=19922945, "4-Axis"=20971521, "5-Axis"=22020097, "6-Axis"=23068673, "7-Axis"=24117249, "LED365"=2684354561, "LED385"=2685403137, "LED440"=2686451713, "LED470"=2687500289, "LED510"=2688548865, "LED540"=2689597441, "LED590"=2690646017, "LED640"=2691694593, "DurchR"=2701131777, "DurchG"=2702180353, "DurchB"=2703228929, "AF"=2704277505, "Laser0"=2717908993, "Laser1"=2718957569, "Laser2"=2720006145, "Laser3"=2721054721, "Servo0"=67108865, "Servo1"=68157441, "Servo2"=69206017, "Servo3"=70254593, "0-TMSI"=100663361, "1-TMSI"=101711937, "x-tmsi"=102760513, "y-tmsi"=103809089, "z-tmsi"=104857665, "orca1"=503316481, "orca2"=503316482, "orca3"=503316483, "orca4"=503316484, "IO-Bank0"=3489660928, "IO-Bank1"=3506438144, ""=0]  # Special-Ticket
  # "command structure, all 4byte ints:\nlength, transfercommand, datalaod\n\ndataload is dependent on  transfercommand:\nWrite: W, offset, data...\nExecute: X\nRead: R, offset, length?\n..."
  n1 = flat-sequence {
    frame #0 {
      # "ohjeh\n...\\Labview\\Colibri\\Drivers\\builds\\SIAM_test_Standalone\\SIAM_test_Standalone.exe\\Drivers\\SIAM\\SIAM_test_Standalone.vi\noder Colibri\\Drivers\\SIAM\\SIAM_test_Standalone.vi"
      # "init"
      n2 = Current VI's Path() -> (path=w5:path)
      n3 = Path To String(path=w5) -> (string=w8:string)
      n4 = call "SplitAtLast.vi"("search char"=".exe", "In-String"=w8) -> ("Front (default)"=w4:string)  [unwired: 1 out]
      n5 = call "SplitAtLast.vi"("search char"=".vi", "In-String"=w4) -> ("Front (default)"=w3:string)  [unwired: 1 out]
      n6 = Concatenate Strings(w3, ".initxml" ("string")) -> (w7:string)
      n7 = String To Path(string=w7) -> (path=w6:path)
      "Ini-file used" <- w6
      n8 = Read from Text File(file (use dialog)=w6) -> (text=w12:string, error out=w11:errorcluster)  [unwired: 3 in, 2 out]
      n9 = case shown="Error" w11 {
        selector: w11 -> [w15 w28]
        tunnel: w12 -> [w16 _]
        tunnel: [w17 w28] -> w10
        frame No Error {
          n10 = call "LvVariantsFromString.vi"("error IO"=w15, "iniString"=w16) -> ("Array"=w14:cluster{"LvVariant":string, "Name":string}[])  [unwired: 8 in, 1 out]
          n11 = for {
            tunnel: w15 -> [w27]
            tunnel: [w21] -> w17
            tunnel: w14 -> [w20] mode=indexing
            n12 = Unbundle(w20) -> ("LvVariant"=w18:string, "Name"=w19:string)
            n13 = invoke class="VI" method="Ctrl Val.Get"(error in=w27, "Control Name"=w19) -> (reference out=w26:refnum<vi>, error out=w23:errorcluster, "Get Control Value Variant"=w25:variant)  [unwired: 2 in, 1 out]
            n14 = Unflatten From XML(xml string=w18, type=w25, error in (no error)=w23) -> (value=w24:variant, error out=w22:errorcluster)
            n15 = invoke class="VI" method="Ctrl Val.Set"(reference=w26, error in=w22, "Control Name"=w19, "Value"=w24) -> (error out=w21:errorcluster)  [unwired: 1 in, 4 out]
          }
        }
        frame Error {
          # "probably no file there"
        }
      }
      "init error" <- w10
    }
  }
  n16 = local write "end-read"(FALSE ("end-read")) -> ()
  n17 = while {
    stop <- "end-read" stop-if-true
    n18 = local read "connection ID"() -> (w30:refnum<k5>)
    n19 = TCP Read(connection ID=w30, bytes to read=4, 7:T13."Buffered" ("mode (standard)"), 9:10 ("timeout ms (25000)")) -> (connection ID out=w34:refnum<k5>, data out=w33:string, error out=w36:errorcluster)  [unwired: 1 in]
    n20 = case shown="No Error" w36 {
      selector: w36 -> [w58 w71]
      tunnel: w33 -> [w62 _]
      tunnel: w34 -> [w59 _]
      tunnel: [w40 w72] -> w37
      frame No Error {
        # "ticket, err, value"
        n21 = Type Cast(type=u32 0, x=w62) -> (*(type *) &x=w52:u32)
        n22 = Multiply(x=w52, y=u32 4) -> (x*y=w50:u32)
        n23 = TCP Read(connection ID=w59, bytes to read=w50, error in (no error)=w58, 7:T13."Buffered" ("mode (standard)"), 9:500 ("timeout ms (25000)")) -> (data out=w56:string, error out=w46:errorcluster)  [unwired: 1 out]
        n24 = String To Byte Array(string=w56) -> (unsigned byte array=w53:u8[])
        n25 = Type Cast(type=i32[] [], x=w53) -> (*(type *) &x=w45:i32[])
        "Return" <- w45
        n26 = call "SIAM-convertReturnToReadable.vi"("Format"="Format", "error in (no error)"=w46, "Return"=w45) -> ("error out"=w41:errorcluster, "CR?"=w48:string, "Readable"=w54:string)  [unwired: 6 out]
        n27 = Index Array(array=w45, index #1=0 ("index"), index #2=2 ("index")) -> (element #1=w43:i32, element #2=w38:i32)
        n28 = Concatenate Strings("return", w54, w48) -> (w55:string)
        n29 = case shown="D0000000" w43 {
          tunnel: w41 -> [w68 w69]
          tunnel: [w66 w69] -> w40
          tunnel: w38 -> [w64 _]
          frame -805306368 {
            n30 = property on="Array" class="Arr (strict)"(error in=w68) -> (error out=w67:errorcluster, "Value"=w65:T5)  [unwired: 1 in, 1 out]
            n31 = call "SIAM-DecodeDigitalReturn.vi"(10:w64, "Array 2"=w65) -> ("Array 3"=w63:T5)  [unwired: 9 in]
            n32 = property on="Array" class="Arr (strict)"(error in=w67, "Value"=w63) -> (error out=w66:errorcluster)  [unwired: 1 in, 1 out]
          }
          frame 0, Default {
          }
        }
        n33 = local write "return"(w55) -> ()
      }
      frame Error {
        w70 = u32 200  # wait after timeout
        # "66=connection closed\n56=timeout\n1=no connection"
        n34 = Unbundle By Name(w71) -> ("code"=w73:i32)
        n35 = case shown="56" w73 {
          tunnel: [w74 errorcluster {"status"=FALSE, "code"=0, "source"=""} ("error out")] -> w72
          tunnel: w71 -> [w74 _]
          frame 1, Default {
            (unwired) FALSE ("Connected")
          }
          frame 56 {
          }
        }
        n36 = Wait (ms)(milliseconds to wait=w70) -> ()  [unwired: 1 out]
      }
    }
    "recieve error" <- w37
  }
  n37 = while {
    stop <- w77 stop-if-true
    n38 = event shown="[8] \"Read\": Value Change" {
      selector: _ -> [_ _ _ _ _ _ _ _ _ _ _ _ _ _ _ _ _ _ _ _]
      dyn-events: _ -> [_ _ _ _ _ _ _ _ _ _ _ _ _ _ _ _ _ _ _ _]
      timeout: "Wait ms" -> [_ _ _ _ _ _ _ _ _ _ _ _ _ _ _ _ _ _ _ _]
      tunnel: [_ _ _ _ _ _ _ _ _ _ _ _ _ _ _ _ _ _ _ "End"] -> w77
      event Timeout {
        n39 = event-data() -> ()  [unwired: 3 out]
        n40 = Array Size(array="direkt command queue") -> (size(s)=w79:i32)
        n41 = Greater Than 0?(x=w79) -> (x > 0?=w78:bool)
        n42 = case shown="True" w78 {
          tunnel: "direkt command queue" -> [_ w85]
          frame False {
            # "no command queued"
          }
          frame True {
            # "start: just set timeout >0"
            n43 = Delete From Array(array=w85, index=0) -> (deleted portion=w84:T17, array with subset deleted=w81:T11)  [unwired: 1 in]
            n44 = local write "direkt command queue"(w81) -> ()
            n45 = Array Size(array=w81) -> (size(s)=w83:i32)
            n46 = Greater Than 0?(x=w83) -> (x > 0?=w82:bool)
            n47 = case shown="True" w82 {
              tunnel: [10000 ("upper limit") w101] -> w90
              tunnel: w81 -> [_ w100]
              frame False {
                # "chek after some s?"
                # "last command"
              }
              frame True {
                # "delay 3ms ..10s"
                # "take next delay"
                n48 = Index Array(array=w100, index=0) -> (element=w93:T17)
                n49 = Unbundle By Name(w93) -> ("Delay 10µs"=w99:u32)
                n50 = Divide(x=w99, y=u32 100) -> (x/y=w97:dbl)
                n51 = To Long Integer(number=w97) -> (32bit integer=w94:i32)
                n52 = In Range and Coerce(upper limit=100000, x=w94, lower limit=3) -> (coerced(x)=w101:i32)  [unwired: 1 out]
              }
            }
            n53 = Build Array(w84) -> (w89:T11)
            n54 = call "SIAM-send.vi"("Script"=w89, "command"=SIAM-send."rundirect" ("special send options")) -> ("error out"=→"send error":errorcluster)  [unwired: 8 in, 1 out]
            n55 = local write "Wait ms"(w90) -> ()
          }
        }
      }
      event "connect": Value Change {
        n56 = event-data() -> ()  [unwired: 6 out]
        n57 = case shown="True" "connect" {
          tunnel: [FALSE w112] -> w102
          frame False {
            # "store ID=0?"
            n58 = local read "connection ID"() -> (w105:refnum<k5>)
            n59 = TCP Close Connection(connection ID=w105) -> (error out=w106:errorcluster)  [unwired: 2 in, 1 out]
            n60 = local write "connect error"(w106) -> ()
          }
          frame True {
            w117 = 0  # Adress
            w119 = u8 73  # Send ID
            # "ticket, err, value"
            # "expect  return\n2,49,0\n49,AE =Wrong Password"
            # "63: no server"
            n61 = local write "recieve error"(errorcluster {"status"=FALSE, "code"=0, "source"=""} ("recieve error")) -> ()
            n62 = String To Byte Array(string="instrument name") -> (unsigned byte array=w116:u8[])
            n63 = Array Size(array=w116) -> (size(s)=w120:i32)
            n64 = TCP Open Connection(address="address", remote port or service name="remote port", timeout ms (60000)=1000) -> (connection ID=w129:refnum<k5>, error out=w110:errorcluster)  [unwired: 1 in, 1 out]
            "connection ID" <- w129
            n65 = Add(x=w120, y=2) -> (x+y=w114:i32)
            n66 = Build Array (concatenate)(w114, w119, w117, w116) -> (w113:i32[])
            n67 = To Unsigned Long Integer(number=w113) -> (unsigned 32bit integer=w121:u32[])
            n68 = Type Cast(x=w121) -> (*(type *) &x=w122:string)  [unwired: 1 in]
            n69 = TCP Write(connection ID=w129, data in=w122, error in (no error)=w110, 9:5000 ("timeout ms (25000)")) -> (connection ID out=w107:refnum<k5>, error out=w111:errorcluster)  [unwired: 1 out]
            n70 = Unbundle By Name(w110) -> ("status"=w127:bool)
            n71 = call "SIAM-send.vi"("connection ID"=w107, "error in (no error)"=w111, "command"=SIAM-send."storeID") -> ("error out"=→"connect error":errorcluster)  [unwired: 7 in, 1 out]
            n72 = Not(x=w127) -> (.not. x?=w112:bool)
          }
        }
        "Connected" <- w102
      }
      event "Special": Value Change {
        n73 = event-data() -> ()  [unwired: 7 out]
        n74 = local read "direkt command queue"() -> (w131:T11)
        n75 = local write "Wait ms"(100 ("Wait for")) -> ()
        n76 = call "SIAM-mergeScripts.vi"("Script 2"="direkt commands", "Script"=w131) -> ("Script out"=w130:T11)  [unwired: 8 in, 1 out]
        n77 = local write "direkt command queue"(w130) -> ()
      }
      event "Clear direct": Value Change {
        n78 = event-data() -> ()  [unwired: 7 out]
        n79 = local write "direkt commands"(T15 [{"Delay 10µs"=0, "command"=4027514895, "P0"=0, "P1"=0, "P2"=0, "P3"=0, "P4"=0, "P5-ticket"=0, ""}] ("direkt commands")) -> ()
      }
      event "Uart-Ascii": Value Change {
        n80 = event-data() -> ()  [unwired: 7 out]
        n81 = call "SIAM-RS232-direkt.vi"("UART: 0..3"="UART: 0..3", "Combo Box"="String") -> ("Script"=w137:T11)  [unwired: 7 in, 2 out]
        n82 = local write "direkt command queue"(w137) -> ()
        n83 = local write "Wait ms"(100 ("Wait for")) -> ()
      }
      event "Uart-TSM": Value Change {
        n84 = event-data() -> ()  [unwired: 7 out]
        n85 = local read "UART: 0..3"() -> (w139:u8)
        n86 = call "SIAM-TML-direkt.vi"("UART: 0..3"=w139, "TSM"="TSM") -> ("Array"=w142:T11)  [unwired: 6 in, 3 out]
        n87 = local write "direkt command queue"(w142) -> ()
        n88 = local write "Wait ms"(100 ("Wait for")) -> ()
      }
      event "Wrapper": Value Change {
        n89 = event-data() -> ()  [unwired: 7 out]
        n90 = call "SIAM-send.vi"("Values"="wrapper[U32]", "command"=SIAM-send."sendValue") -> ("error out"=w143:errorcluster)  [unwired: 8 in, 1 out]
        n91 = local write "connect error"(w143) -> ()
      }
      event "Array": Value Change {
        n92 = event-data() -> ("OldVal"=w147:T5, "NewVal"=w146:T5)  [unwired: 5 out]
        n93 = for {
          tunnel: w147 -> [w150] mode=indexing
          tunnel: w146 -> [w148] mode=indexing
          n94 = Not Equal?(x=w150, y=w148) -> (x != y?=w149:bool)
          n95 = case shown="True" w149 {
            tunnel: w148 -> [_ w156]
            frame False {
            }
            frame True {
              w158 = T8 3489660929 items=["read_x-Motor_status_ticket"=17305600, "init_x-Motor"=17760263, "read_x-Motor_absolute_ticket"=16781312, "move_x-Motor_absolute"=16777217, "move_x-Motor_relative"=16842753, "read_y-Motor_status_ticket"=18354176, "init_y-Motor"=18808839, "read_y-Motor_absolute_ticket"=17829888, "move_y-Motor_absolute"=17825793, "move_y-Motor_relative"=17891329, "read_z-Motor_status_ticket"=19402752, "init_z-Motor"=19857415, "stop_z-Motor"=19857423, "start_z-Motor"=19857422, "read_z-Motor_absolute_ticket"=18878464, "move_z-Motor_absolute"=18874369, "move_z-Motor_relative"=18939905, "read_Objective_status_ticket"=20451328, "init_Objective"=20905991, "read_Objective_absolute_ticket"=19927040, "move_Objective_absolute"=19922945, "move_Objective_relative"=19988481, "read_Filter_status_ticket"=21499904, "init_Filter"=21954567, "read_Filter_absolute_ticket"=20975616, "move_Filter_absolute"=20971521, "move_Filter_relative"=21037057, "read_Trans-Rad_status_ticket"=22548480, "init_Trans-Rad"=23003143, "read_Trans-Rad_absolute_ticket"=22024192, "move_Trans-Rad_absolute"=22020097, "move_Trans-Rad_relative"=22085633, "read_FRET_status_ticket"=23597056, "init_FRET"=24051719, "read_FRET_absolute_ticket"=23072768, "move_FRET_absolute"=23068673, "move_FRET_relative"=23134209, "read_SI-Rad_status_ticket"=24645632, "init_SI-Rad"=25100295, "read_SI-Rad_absolute_ticket"=24121344, "move_SI-Rad_absolute"=24117249, "move_SI-Rad_relative"=24182785, "end_no_ticket"=4027514895, "end_ticket"=4027518991, "IO-read_bank0"=3489665024, "IO-write_bank0"=3489660929, "IO-read_bank1"=3506442240, "IO-write_bank1"=3506438145, "Analog-write_DA0-0"=2684354561, "Analog-write_DA0-1"=2685403137, "Analog-write_DA0-2"=2686451713, "Analog-write_DA0-3"=2687500289, "Analog-write_DA0-4"=2688548865, "Analog-write_DA0-5"=2689597441, "Analog-write_DA0-6"=2690646017, "Analog-write_DA0-7"=2691694593, "Analog-write_DA1-0"=2701131777, "Analog-write_DA1-1"=2702180353, "Analog-write_DA1-2"=2703228929, "Analog-write_DA1-3"=2704277505, "Analog-write_DA1-4"=2705326081, "Analog-write_DA1-5"=2706374657, "Analog-write_DA1-6"=2707423233, "Analog-write_DA1-7"=2708471809, "Analog-read_AD0-0"=2818576384, "Analog-read-store_AD0-0"=2818572290, "IO-delay_bank0"=3489923073, "IO-delay_bank0_fromVar"=3489923075, "read_cam_clock"=3289124864, "store_cam_clock"=3289120770, "read_cam_phase"=3289190400, "set_cam_deadtime"=3288989697, "set_cam_10uscycles"=3289055233, "set_cam_10uscycles_fromVariable"=3289055235, "calc_cam"=3289317386, "store_cam_Var"=3289251842, "math_addToVariable"=4060086278, "readVar"=4060090368, "writeVar"=4060086273, "copyVar"=4060086276, "decrement_branchRel_if_equal"=4043374945, "decrement_branchRel_if_greaterequal"=4043375201, "decrement_branchRel_if_greaterequal_withTicket"=4043379297, "decrement_branchRel_if_smaller"=4043375457, "increment_branchRel_if_smaller"=4043375473, "set_1Galvo"=101712113, "set_x-Galvo"=102760689, "set_y-Galvo"=103809265, "set_z-Fokus"=104857841, "set_1Galvo_position-only"=101711937, "set_x-Galvo_position-only"=102760513, "set_y-Galvo_position-only"=103809089, "set_z-Fokus_position-only"=104857665, "set_x-Galvo_position-only_ticket"=102764609, "set_y-Galvo_position-only_ticket"=103813185, "set_z-Fokus_position-only_ticket"=104861761, "set_x-Galvo_relativ-only"=102760577, "set_y-Galvo_relativ-only"=103809153, "set_z-Fokus_relativ-only"=104857729, "set_x-Galvo_speed-only"=102760481, "set_y-Galvo_speed-only"=103809057, "set_z-Fokus_speed-only"=104857633, "read_1Galvo_ticket"=101716032, "read_x-Galvo_ticket"=102764608, "read_y-Galvo_ticket"=103813184, "read_z-Focus_ticket"=104861760, "x-Galvo_pos_fromVar"=102760515, "y-Galvo_pos_fromVar"=103809091, "z-Focus_pos_fromVar"=104857667, "Servo0"=67108865, "Servo1"=68157441, "Servo2"=69206017] ("Device")
              n96 = Unbundle(w156) -> ("Digital-out"=w155:T18, "Boolean"=w154:bool)
              n97 = Boolean To (0,1)(Boolean=w154) -> (0, 1=w161:i16)
              n98 = To Unsigned Long Integer(number=w161) -> (unsigned 32bit integer=w157:u32)
              n99 = Logical Shift(y=w155, x=u32 1) -> (x << y=w160:u32)
              n100 = Logical Shift(y=w155, x=w157) -> (x << y=w159:u32)
              n101 = Bundle By Name(cluster=T16 {"rel 10µs"=0, "Device"=3489660929, "data0"=0, "data1"=0, "data2"=0, "data3"=0, "data4"=0, "data5"=0, "direct"} ("output cluster"), "Device"=w158, "data0"=w160, "data1"=w159) -> (w153:T16)
              n102 = Build Array(w153) -> (w152:T19)
              n103 = local write "Send debug"(w152) -> ()
              n104 = call "SIAM-send.vi"("Script"=w152, "command"=SIAM-send."rundirect") -> ("error out"=w151:errorcluster)  [unwired: 8 in, 1 out]
              n105 = local write "send error"(w151) -> ()
            }
          }
        }
      }
      event "Read": Value Change {
        w166 = T2 3489660928 items=["255Axis"=16777217, "1-Axis"=17825793, "2-Axis"=18874369, "3-Axis"=19922945, "4-Axis"=20971521, "5-Axis"=22020097, "6-Axis"=23068673, "7-Axis"=24117249, "LED365"=2684354561, "LED385"=2685403137, "LED440"=2686451713, "LED470"=2687500289, "LED510"=2688548865, "LED540"=2689597441, "LED590"=2690646017, "LED640"=2691694593, "DurchR"=2701131777, "DurchG"=2702180353, "DurchB"=2703228929, "AF"=2704277505, "Laser0"=2717908993, "Laser1"=2718957569, "Laser2"=2720006145, "Laser3"=2721054721, "Servo0"=67108865, "Servo1"=68157441, "Servo2"=69206017, "Servo3"=70254593, "0-TMSI"=100663361, "1-TMSI"=101711937, "x-tmsi"=102760513, "y-tmsi"=103809089, "z-tmsi"=104857665, "orca1"=503316481, "orca2"=503316482, "orca3"=503316483, "orca4"=503316484, "IO-Bank0"=3489660928, "IO-Bank1"=3506438144, ""=0]  # Special-Ticket
        n106 = event-data() -> ()  [unwired: 7 out]
        n107 = Bundle By Name(cluster=T16 {"rel 10µs"=0, "Device"=3489665024, "data0"=0, "data1"=0, "data2"=0, "data3"=0, "data4"=0, "data5"=0, "direct"} ("output cluster"), "data0"=-1, "data5"=w166) -> (w167:T16)
        n108 = Build Array(w167) -> (w168:T19)
        n109 = call "SIAM-send.vi"("Script"=w168, "command"=SIAM-send."rundirect") -> ()  [unwired: 8 in, 2 out]
      }
      event "SendScript": Value Change {
        n110 = event-data() -> ()  [unwired: 7 out]
        n111 = call "SIAM-send.vi"("Script"="Script", "command"=SIAM-send."sendlist") -> ()  [unwired: 8 in, 2 out]
      }
      event "Run": Value Change {
        n112 = event-data() -> ()  [unwired: 7 out]
        n113 = call "SIAM-send.vi"("command"=SIAM-send."run") -> ()  [unwired: 9 in, 2 out]
      }
      event "Save": Value Change {
        n114 = event-data() -> ()  [unwired: 7 out]
        n115 = local read "Script"() -> (w175:T11)
        n116 = call "SIAMScript_to_String.vi"("Script"=w175) -> ("String"=w174:string)  [unwired: 9 in, 1 out]
        n117 = Write to Text File(text=w174) -> ()  [unwired: 3 in, 3 out]
      }
      event "Load": Value Change {
        n118 = event-data() -> ()  [unwired: 7 out]
        n119 = Read from Text File(prompt (Open existing file)="Select File") -> (text=w177:string, error out=w176:errorcluster)  [unwired: 3 in, 2 out]
        n120 = case shown="No Error" w176 {
          selector: w176 -> [w179 _]
          tunnel: w177 -> [w180 _]
          frame No Error {
            n121 = call "ImportSIAMScript.vi"("error in (no error)"=w179, "String"=w180) -> ("Script"=w181:T20)  [unwired: 8 in, 1 out]
            n122 = local write "Script"(w181) -> ()
          }
          frame Error {
          }
        }
      }
      event "Calculate SIM": Value Change {
        n123 = event-data() -> ()  [unwired: 7 out]
        n124 = call "SIAM-SIMStack_v3.vi"("Constants"="Constants", "User"="User") -> ("SIAMScript"=w185:T11, "Camera"=→"Camera":T7)  [unwired: 7 in, 1 out]
        n125 = local write "Script"(w185) -> ()
      }
      event "Axis": Value Change {
        # "block frontpanel!"
        n126 = event-data() -> ("OldVal"=w189:T4, "NewVal"=w188:T4)  [unwired: 5 out]
        n127 = Cluster To Array(cluster=w189) -> (array=w186:cluster{"Axis-Ring":T2, "Position":i32}[])
        n128 = Cluster To Array(cluster=w188) -> (array=w187:cluster{"Axis-Ring":T2, "Position":i32}[])
        n129 = for {
          tunnel: w186 -> [w193] mode=indexing
          tunnel: w187 -> [w192] mode=indexing
          n130 = Not Equal?(x=w193, y=w192) -> (x != y?=w191:bool)
          n131 = case shown="True" w191 {
            tunnel: w192 -> [_ w203]
            frame False {
            }
            frame True {
              # "sorry direct too fast\nwork with Direkt list?"
              n132 = local read "direkt command queue"() -> (w197:T11)
              n133 = local read "TSM"() -> (w200:T12)
              n134 = Unbundle(w203) -> ("Axis-Ring"=w202:T2, "Position"=w201:i32)
              n135 = Unbundle By Name(w200) -> ("RS232-axis"=w199:u8)
              n136 = call "Axis-To-SIAM-direkt.vi"("Extra Information"=w199, "Position"=w201, "Axis-Ring"=w202) -> ("Direct Commands"=w196:T11)  [unwired: 7 in, 1 out]
              "Send debug" <- w196
              n137 = call "SIAM-mergeScripts.vi"("Enum"=enum16{"Append", "try merge"}."Append", "Script 2"=w196, "Script"=w197) -> ("Script out"=w195:T11)  [unwired: 7 in, 1 out]
              n138 = local write "direkt command queue"(w195) -> ()
              n139 = local write "Wait ms"(10 ("Wait ms")) -> ()
            }
          }
        }
        n140 = Wait (ms)(milliseconds to wait=u32 100) -> ()  [unwired: 1 out]
      }
      event "New Ini": Value Change {
        # "flatten to string"
        n141 = event-data() -> ()  [unwired: 7 out]
        n142 = Current VI's Path() -> (path=w215:path)
        n143 = Path To String(path=w215) -> (string=w217:string)
        n144 = call "SplitAtLast.vi"("search char"=".exe", "In-String"=w217) -> ("Front (default)"=w213:string)  [unwired: 1 out]
        n145 = call "SplitAtLast.vi"("search char"=".vi", "In-String"=w213) -> ("Front (default)"=w212:string)  [unwired: 1 out]
        n146 = Concatenate Strings(w212, ".initxml" ("string")) -> (w216:string)
        n147 = String To Path(string=w216) -> (path=w204:path)
        n148 = Read from Text File(file (use dialog)=w204) -> (refnum out=w206:refnum<file>, text=w210:string, error out=w211:errorcluster)  [unwired: 3 in, 1 out]
        n149 = case shown="Error" w211 {
          selector: w211 -> [w226 _]
          tunnel: w210 -> [w230 _]
          tunnel: [w227 w237] -> w209
          tunnel: [w225 w236] -> w205
          frame No Error {
            # "update existing entries"
            n150 = call "LvVariantsFromString.vi"("error IO"=w226, "iniString"=w230) -> ("error out"=w228:errorcluster, "Array"=w229:cluster{"LvVariant":string, "Name":string}[])  [unwired: 8 in]
            n151 = for {
              tunnel: w229 -> [w235] mode=indexing
              tunnel: w228 -> [w233]
              tunnel: [w232] -> w227 mode=indexing
              tunnel: [w231] -> w225
              # "ignore errors!"
              n152 = Unbundle(w235) -> ("Name"=w234:string)  [unwired: 1 out]
              n153 = invoke class="VI" method="Ctrl Val.Get"(error in=w233, "Control Name"=w234) -> (error out=w231:errorcluster, "Get Control Value Variant"=w232:variant)  [unwired: 2 in, 2 out]
            }
          }
          frame Error {
            # "all new"
            n154 = invoke class="VI" method="Ctrl Val.Get All"("Controls"=TRUE) -> (error out=w236:errorcluster, "Get All Control Values Variant"=w238:cluster{"Name":string, "Variant Data":variant}[])  [unwired: 3 in, 2 out]
            n155 = for {
              tunnel: w238 -> [w241] mode=indexing
              tunnel: [w240] -> w237 mode=indexing
              n156 = Unbundle By Name(w241) -> ("Variant Data"=w240:variant)
            }
          }
        }
        n157 = Close File(refnum=w206) -> ()  [unwired: 1 in, 2 out]
        n158 = local write "init error"(w205) -> ()
        n159 = for {
          shift-right: [w221] -> w207
          shift-left: "" -> [w224]
          tunnel: w209 -> [w220] mode=indexing
          n160 = Flatten To XML(anything=w220) -> (xml string=w223:string)
          n161 = Concatenate Strings(w224, w223, "\r\n") -> (w221:string)
        }
        n162 = Write to Text File(file (use dialog)=w204, text=w207) -> ()  [unwired: 2 in, 3 out]
      }
      event "Clear": Value Change {
        n163 = event-data() -> ()  [unwired: 7 out]
        n164 = case shown="False" "Clear" {
          frame False {
          }
          frame True {
            n165 = local write "return"("") -> ()
          }
        }
      }
      event "ClearScript": Value Change {
        n166 = event-data() -> ()  [unwired: 7 out]
        n167 = local write "Script"(T15 [] ("Script")) -> ()
      }
      event "xy": Value Change {
        n168 = event-data() -> ("OldVal"=w257:T6, "NewVal"=w256:T6)  [unwired: 5 out]
        n169 = Not Equal?(x=w257, y=w256) -> (x != y?=w255:T6)
        n170 = property on="Axis" class="Clust (strict)"() -> ("Value"=w247:T4)  [unwired: 2 in, 2 out]
        n171 = Unbundle(w255) -> ("x"=w254:bool, "-x"=w251:bool, "-y"=w252:bool)  [unwired: 1 out]
        n172 = Or(x=w251, y=w252) -> (x .or. y?=w250:bool)
        n173 = Or(x=w254, y=w251) -> (x .or. y?=w253:bool)
        n174 = Negate(x="step") -> (-x=w248:i32)
        n175 = Select(t=w248, s=w250, f="step") -> (s? t:f=w246:i32)
        n176 = case shown="True" w253 {
          tunnel: [w261 w265] -> w245
          tunnel: w247 -> [w260 w266]
          tunnel: w246 -> [w262 w267]
          frame False {
            # "y"
            n177 = Unbundle By Name(w260) -> ("Linear.Position"=w259:i32)
            n178 = Add(x=w259, y=w262) -> (x+y=w258:i32)
            n179 = Bundle By Name(cluster=w260, "Linear.Position"=w258) -> (w261:T4)
          }
          frame True {
            # "x"
            n180 = Unbundle By Name(w266) -> ("Linear.Position"=w264:i32)
            n181 = Add(x=w264, y=w267) -> (x+y=w263:i32)
            n182 = Bundle By Name(cluster=w266, "Linear.Position"=w263) -> (w265:T4)
          }
        }
        n183 = property on="Axis" class="Clust (strict)"("Val(Sgnl)"=w245) -> ()  [unwired: 2 in, 2 out]
      }
      event "End": Value Change {
        n184 = event-data() -> ()  [unwired: 7 out]
        n185 = local read "connection ID"() -> (w269:refnum<k5>)
        n186 = TCP Close Connection(connection ID=w269) -> (error out=w271:errorcluster)  [unwired: 1 in, 2 out]
        n187 = local write "Connected"(FALSE ("Connected")) -> ()
        n188 = local write "connect error"(w271) -> ()
        n189 = disable-structure shown="Disabled" {
          frame Disabled {
            n190 = invoke class="VI" method="FP.Close"() -> ()  [unwired: 3 in, 3 out]
          }
          frame Enabled {
          }
        }
        n191 = local write "end-read"("End") -> ()
      }
    }
  }
